vi "uA_Measurement_kit_Logging.vi"() -> ()   [LabVIEW 2017]
uses:
  Range_Shunt_selector.ctl
  <vilib>/Waveform/WDTFileIO.llb/ Write Waveform to File.vi
  <vilib>/Utility/file.llb/Write Delimited Spreadsheet (string).vi
  <vilib>/Waveform/WDTFileIO.llb/Read Waveform from File.vi
  <vilib>/Utility/config.llb/Write Key (I32).vi
  <vilib>/Utility/config.llb/Write Key (Boolean).vi
  <vilib>/Utility/config.llb/Read Key (I32).vi
  <vilib>/Utility/config.llb/Read Key (Boolean).vi
  <vilib>/measure/madcrms.llb/Basic Averaged DC-RMS for 1 Chan.vi
  <resource>/objmgr/daqmx.rc
  <vilib>/Utility/config.llb/NI_LVConfig.lvlib
  <vilib>/measure/NI_MAPro.lvlib
panel:
  out "First_time":timestamp
  out "Ver":string
  out "appended path":path
  out "current time":timestamp
  out "Samples":i32=20000
  out "error out 3":errorcluster
  out "PhysicalChanName":tag
  out "DEV SN":u32 format="%.0x"
  out "mARange":dbl
  out "Boolean":bool
  out "DevSerialNum":u32
  in  "uA_bank0":dbl=1.5 format="%#_13g"
  out "Task out":refnum<k21>="Stop"
  out "Sample rate":dbl=20000.0 format="%#_13g"
  out "Clear":bool=TRUE
  out "seconds since 1Jan1904":timestamp
  in  "Tab Control":enum32{"Current Tracking", "Logging"}(tab)
  out "String":string
  out "Save":bool
  out "Total Time":i32 format="%<%H:%M:%S>t "
  in  "Sampling Rate":T1(ring)
  out "out_range":bool
  in  "Save setting":bool
  out "PW_Source":bool
  out "EX_IN_INdicator":bool
  out "Lable.Unit_VOl_MA_UA":string
  in  "Ext PW Vol Monitor":bool
  out "POWER ON_OFF":bool
  out "vbat_lb":dbl format="%#_4f"
  in  "bypass Shunt":bool
  in  "Internal PW":bool
  in  "USB":tag="Dev1"
  out "schematic":bool
  in  "Save":bool
  in  "Load":bool
  in  "Calib":bool
  in  "Power ON/OFF":bool
  in  "Profile":enum16{"SAM", "DIANA", "Hi-POWER", "Other..."}(ring)
  in  "Take Picture":bool
  in  "Orginal":bool
  in  "Clear Graph":bool
  in  "ZOOM M1M2":bool
  in  "ZOOM -":bool
  in  "ZOOM +":bool
  in  "stop":bool
  out "Vbat":dbl format="%#.3f"
  in  "Measure":bool
  in  "Range - Shunts":T2
  out "PW_Internal_Source":dbl
  out "Min":dbl
  out "Max":dbl
  out "Delta(s)":sgl
  in  "Center":bool
  out "Avg":dbl
  out "Waveform_main":waveform(sgl)(graph)
  out "Waveform_sub":waveform(dbl)(graph)
  out "Average (uA)":dbl caption="Average (mA)" format="%#_6f"
  in  "Vout  - Vbat profile":enum16{"3.8VDC", "2.9VDC", "By Pass", "4.0VDC"}(ring)=enum."2.9VDC" caption="Vout  - Vbat"
  # "Vbat"
  # "Vdut- Vbat"
  # "DUT"
  # "µPower kit for Wear OS Dev"
  # "Rs"
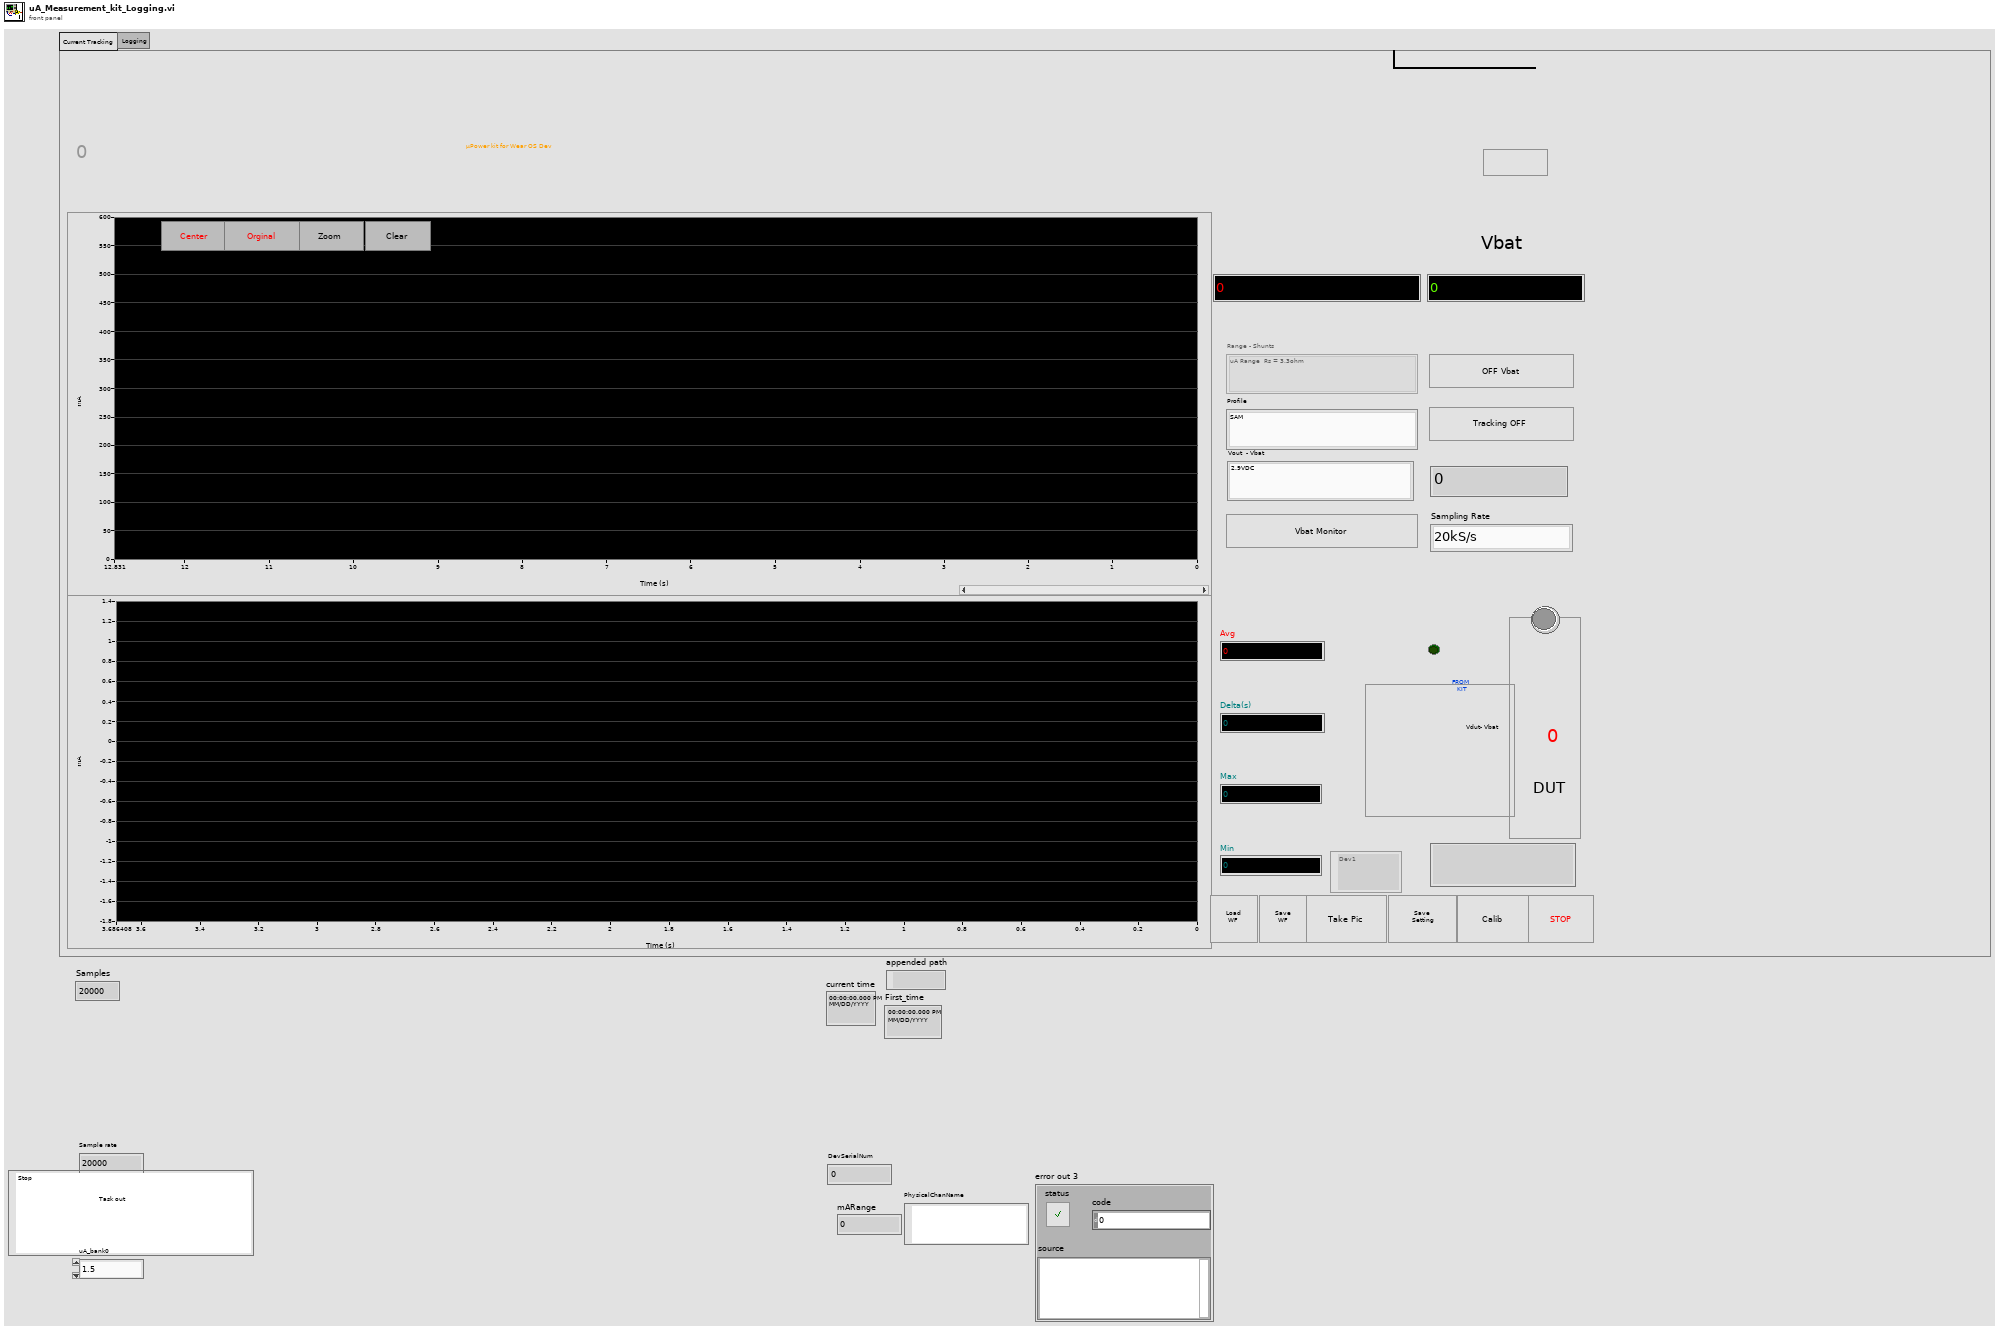
[diagram p1: front panel]
types:
  T1 = enum16{"20kS/s", "10kS/s", "5kS/s", "2kS/s", "1kS/s", "500S/s", "100S/s"}
  T2 = typedef "Range_Shunt_selector.ctl" = enum16{"uA Range  Rs = 3.3ohm", "mA Range Rs = 3.3ohm", "mA Range Rs = 1ohm", "mA Range Rs = 1ohm - X2"}
  T3 = enum8{"Enabled", "Disabled", "Disabled and Grayed Out"}
  T4 = enum16{"open", "replace", "create", "open or create", "replace or create", "replace or create with confirmation"}
  T5 = typedef "NI_LVConfig.lvlib/Config Data RefNum.ctl" = refnum<k1>
  T6 = enum16{"Internal PW Source", "External PW Source"}
  T7 = enum16{"Turn On bypass - Off Shunt", "Turn Off bypass - On Shunt"}
  T8 = typedef "LVCursorListTypeDef.ctl" = cluster{"Name":string, "Color":u32, "Style":u8, "Point Style":u8, "Name Visible":bool, "Allow Drag":bool, "Cursor Mode":u32, "Plot":i32, "Index":i32, "Position":cluster{"X":dbl, "Y":dbl}, "X Scale":u32, "Y Scale":u32, "Watch Plots":i32[], "Watch All Plots":bool, "Plot Area":i32, "Label Offset":cluster{"X":dbl, "Y":dbl}}[]
  T9 = typedef "imagedata.ctl" = cluster{"image type":i32, "image depth":i32, "image":u8[], "mask":u8[], "colors":u32[], "Rectangle":cluster{"left":i16, "top":i16, "right":i16, "bottom":i16}}
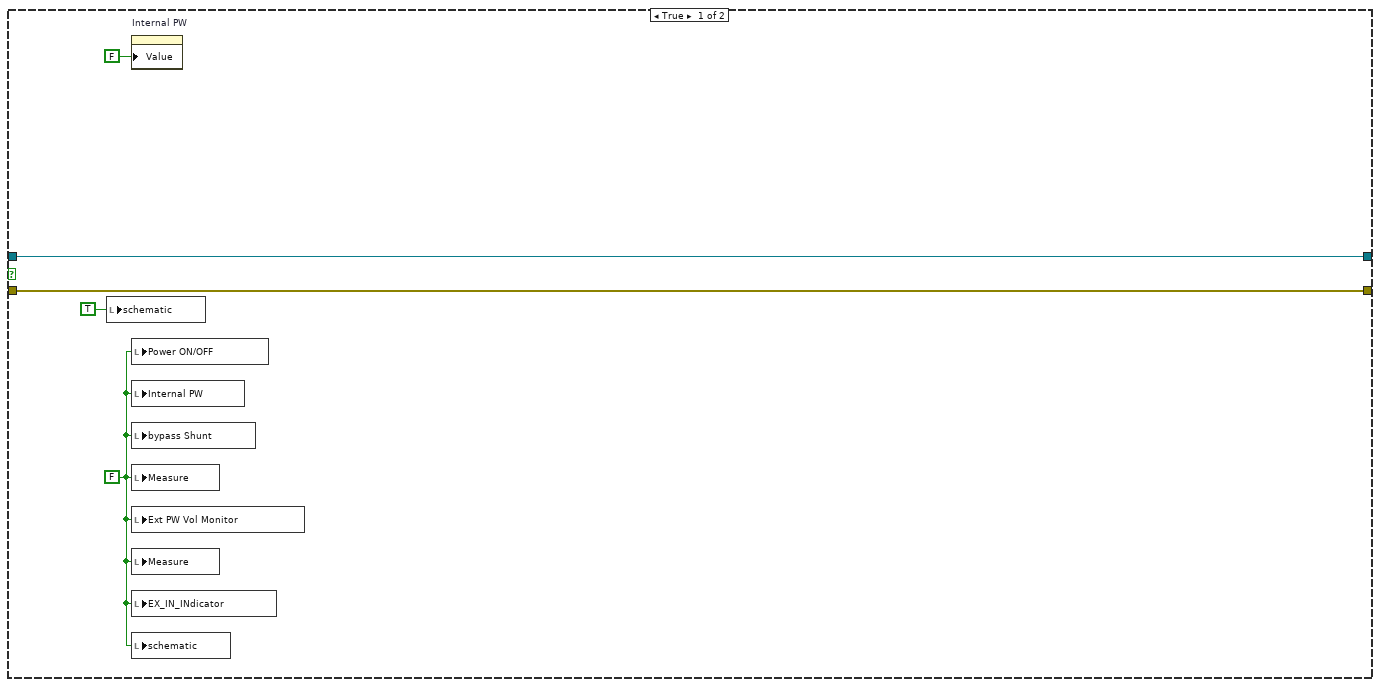
[diagram p3: hidden frame]
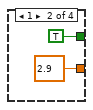
[diagram p4: hidden frame]
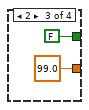
[diagram p5: hidden frame]
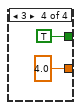
[diagram p6: hidden frame]
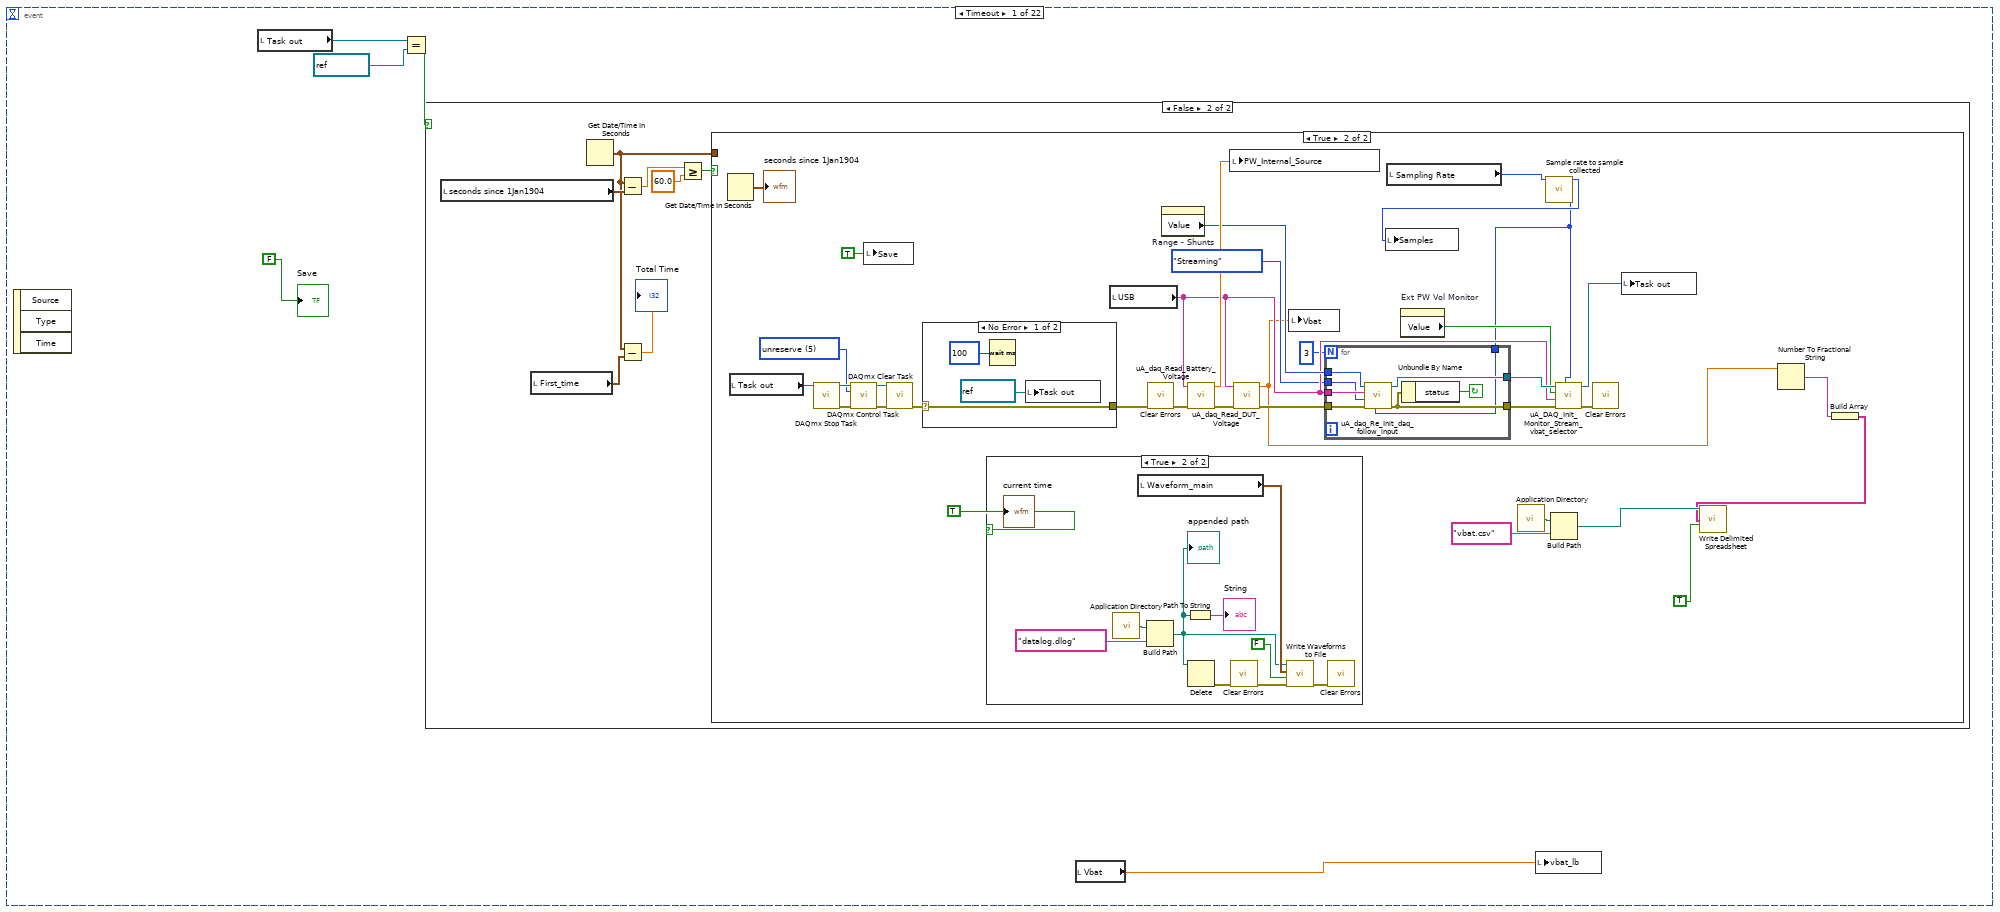
[diagram p8: hidden frame]
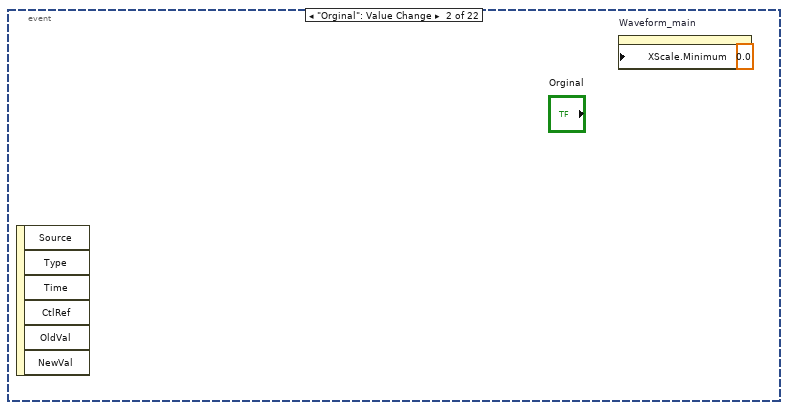
[diagram p13: hidden frame]
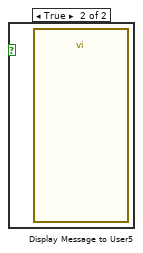
[diagram p14: hidden frame]
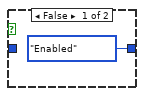
[diagram p15: hidden frame]
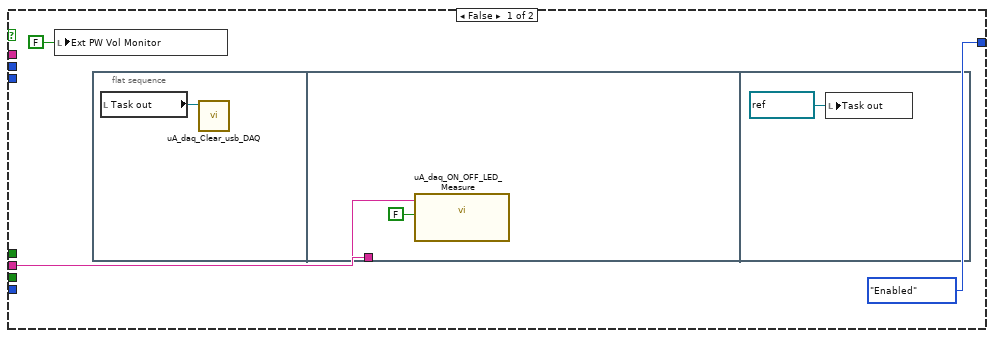
[diagram p16: hidden frame]
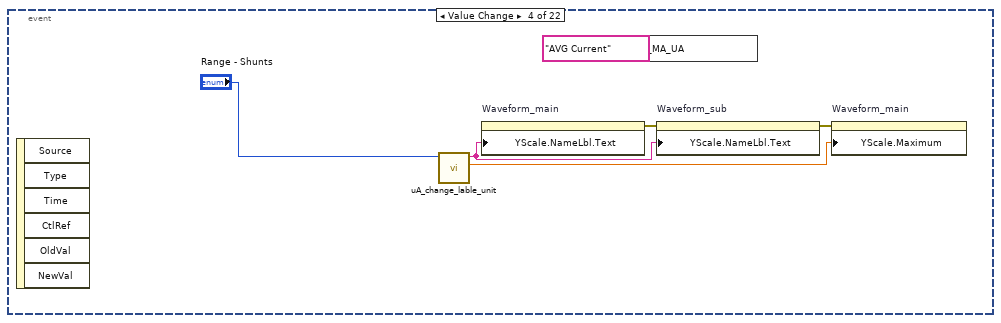
[diagram p17: hidden frame]
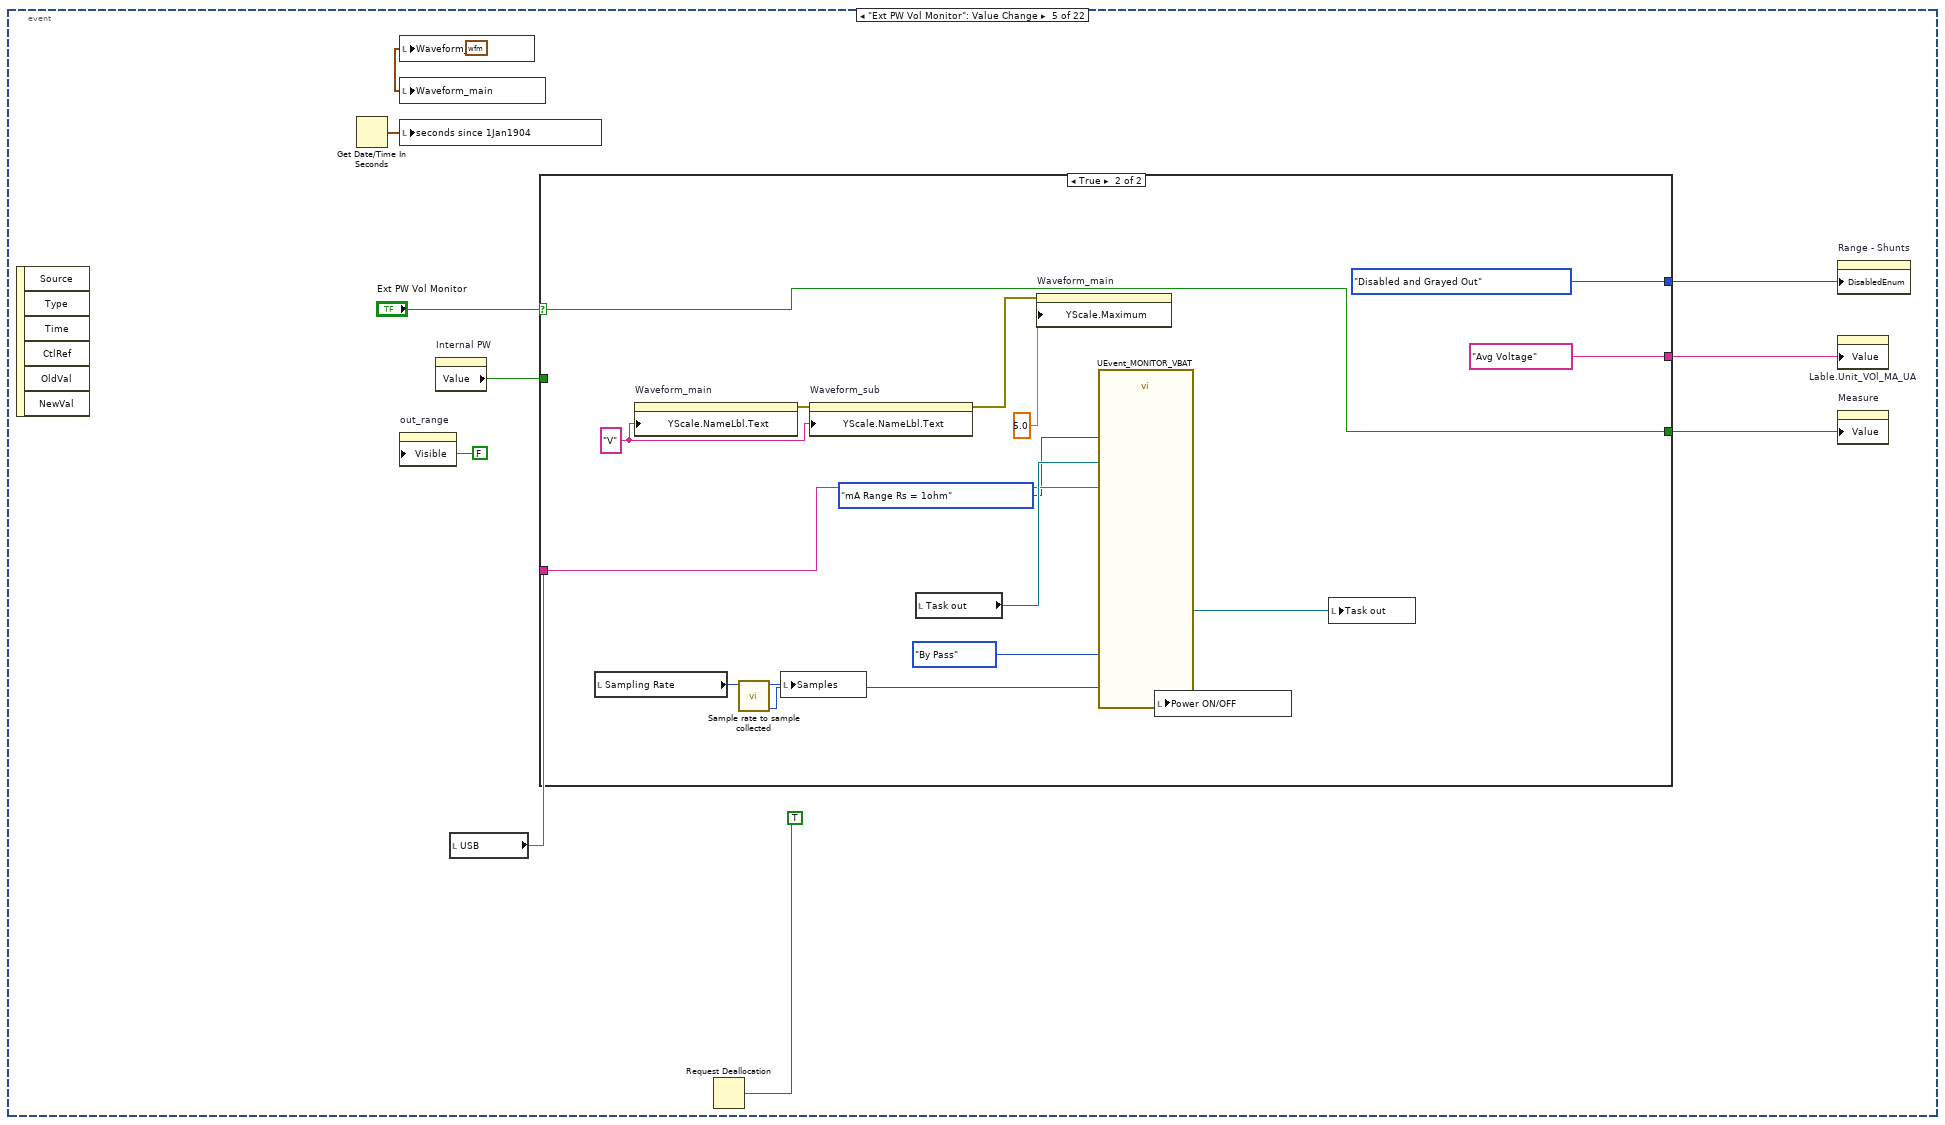
[diagram p18: hidden frame]
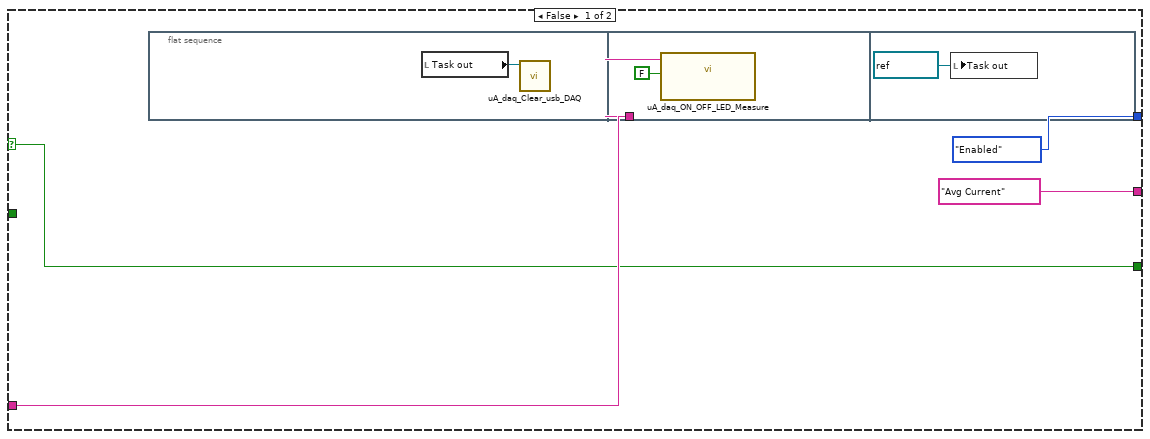
[diagram p19: hidden frame]
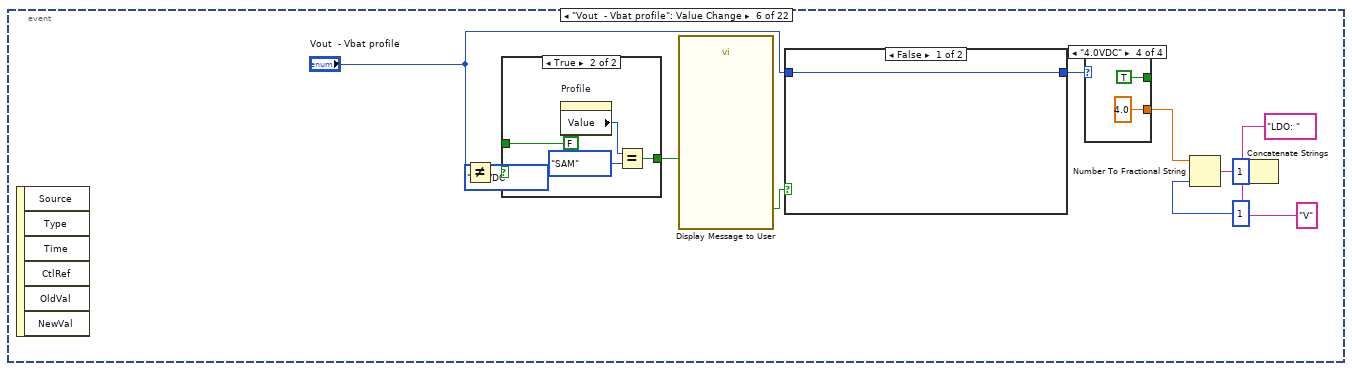
[diagram p20: hidden frame]
diagram:
  w2 = 24164516  # 1200s
  n1 = flat-sequence {
    tunnel: [w45] -> w5
    tunnel: [w48] -> w4
    frame #0 {
      w15 = TRUE ("s")
      w26 = FALSE ("Power ON/OFF")
      w45 = refnum<k21> "Stop" ("task out")
      n2 = property class="DAQmx System"() -> (error out=w39:errorcluster, "Device Names"=w40:tag[])  [unwired: 2 in, 1 out]
      n3 = property on="Range - Shunts" class="Enum (strict)"("DisabledEnum"=T3."Enabled" ("Disabled")) -> (error out=w8:errorcluster)  [unwired: 2 in, 1 out]
      n4 = local write "Vout  - Vbat profile"(enum16{"3.8VDC", "2.9VDC", "By Pass", "4.0VDC"}."By Pass" ("Vout  - Vbat profile")) -> ()
      n5 = local write "Profile"(enum16{"SAM", "DIANA", "Hi-POWER", "Other..."}."Hi-POWER" ("Profile")) -> ()
      n6 = for {
        tunnel: w40 -> [w102] mode=indexing
        shift-right: [w106] -> _
        shift-left: w39 -> [w107]
        tunnel: [w102] -> w38
        tunnel: [w101] -> w20
        stop <- w103 stop-if-true
        n7 = property class="DAQmx Device"(error in=w107, "Active Device"=w102) -> (error out=w106:errorcluster, "DevSerialNum"=w101:u32, "DevIsSimulated"=w105:bool)  [unwired: 1 in, 1 out]
        n8 = Equal?(x=w105, y=FALSE) -> (x = y?=w103:bool)
      }
      "DEV SN" <- w20
      n9 = local write "Power ON/OFF"(w26) -> ()
      n10 = local write "POWER ON_OFF"(w26) -> ()
      n11 = Select(t="Average (mA)" ("Caption.Text"), s=w15, f="Average (uA)" ("Caption.Text")) -> (s? t:f=w18:string)
      n12 = call <vilib>:"Application Directory.vi"() -> ("Application Directory"=w33:path)
      n13 = Select(t="mA" ("Caption.Text"), s=w15, f="uA" ("Caption.Text")) -> (s? t:f=w17:string)
      n14 = property on="out_range" class="Bool (strict)"(error in=w8, "Visible"=FALSE) -> (error out=w11:errorcluster)  [unwired: 1 in, 1 out]
      n15 = Build Path(base path=w33, name or relative path="Setting.cfg") -> (appended path=w31:path)
      n16 = property on="Average (uA)" class="DigNum (strict)"("Caption.Text"=w18) -> ()  [unwired: 2 in, 2 out]
      n17 = property on="Waveform_sub" class="WFGraph (strict)"("YScale.NameLbl.Text"=w17) -> ()  [unwired: 2 in, 2 out]
      n18 = property on="Waveform_main" class="WFGraph (strict)"("YScale.NameLbl.Text"=w17) -> ()  [unwired: 2 in, 2 out]
      n19 = call <vilib>:"Open Config Data.vi"("configuration file path"=w31) -> ("error out"=w27:errorcluster, "file created?"=w34:bool, "refnum"=w30:T5)  [unwired: 8 in]
      n20 = property on="Ext PW Vol Monitor" class="Bool (strict)"(error in=w11, "Value"=FALSE ("Record uA & Vbat")) -> (error out=w10:errorcluster)  [unwired: 1 in, 1 out]
      n21 = case shown="False" w34 {
        tunnel: w27 -> [w62 w92]
        tunnel: [w62 w87] -> w28
        tunnel: [w61 w86] -> w29
        tunnel: w30 -> [w61 w75]
        frame True {
          w60 = FALSE ("Measure")
          n22 = local write "schematic"(TRUE ("schematic")) -> ()
          n23 = property on="Internal PW" class="Bool (strict)"("Value"=FALSE ("Internal PW")) -> ()  [unwired: 2 in, 2 out]
          n24 = local write "Power ON/OFF"(w60) -> ()
          n25 = local write "Internal PW"(w60) -> ()
          n26 = local write "bypass Shunt"(w60) -> ()
          n27 = local write "Measure"(w60) -> ()
          n28 = local write "Ext PW Vol Monitor"(w60) -> ()
          n29 = local write "Measure"(w60) -> ()
          n30 = local write "EX_IN_INdicator"(w60) -> ()
          n31 = local write "schematic"(w60) -> ()
        }
        frame False {
          (unwired) FALSE ("Visible")
          w63 = TRUE
          w76 = "SETTING" ("section")
          n32 = Not(x=w63) -> ()  [unwired: 1 out]
          n33 = local write "Internal PW"(w63) -> ()
          n34 = local write "EX_IN_INdicator"(w63) -> ()
          n35 = local write "Vout  - Vbat profile"(enum16{"3.8VDC", "2.9VDC", "By Pass", "4.0VDC"}."By Pass" ("Vout  - Vbat profile")) -> ()
          n36 = local write "Profile"(enum16{"SAM", "DIANA", "Hi-POWER", "Other..."}."Hi-POWER" ("Profile")) -> ()
          n37 = call-poly <vilib>:"Read Key.vi"("section"=w76, "error in (no error)"=w92, "key"="Range - Shunts", "refnum"=w75) -> ("error out"=w91:errorcluster, "refnum out"=w78:T5)  [unwired: 4 in, 2 out]
          n38 = local write "Range - Shunts"(Range_Shunt_selector."mA Range Rs = 1ohm" ("Range - Shunts")) -> ()
          n39 = call-poly <vilib>:"Read Key.vi"("section"=w76, "error in (no error)"=w91, "key"="Profile", "refnum"=w78) -> ("error out"=w90:errorcluster, "refnum out"=w77:T5)  [unwired: 4 in, 2 out]
          n40 = call-poly <vilib>:"Read Key.vi"("section"=w76, "error in (no error)"=w90, "key"="Vout  - Vbat profile", "refnum"=w77) -> ("error out"=w89:errorcluster, "value"=w67:i32, "refnum out"=w79:T5)  [unwired: 4 in, 1 out]
          n41 = case shown="0, Default" w67 {
            tunnel: [3.8 2.9 99.0 4.0] -> w71
            tunnel: [TRUE ("Visible") TRUE ("Visible") FALSE ("Visible") TRUE ("Visible")] -> _
            frame 0, Default {
            }
            frame 1 {
            }
            frame 2 {
            }
            frame 3 {
            }
          }
          n42 = call-poly <vilib>:"Read Key.vi"("section"=w76, "error in (no error)"=w89, "key"="Internal PW", "refnum"=w79) -> ("error out"=w88:errorcluster, "refnum out"=w80:T5)  [unwired: 4 in, 2 out]
          n43 = call-poly <vilib>:"Read Key.vi"("section"=w76, "error in (no error)"=w88, "key"="bypass Shunt", "refnum"=w80) -> ("error out"=w87:errorcluster, "value"=w74:bool, "refnum out"=w86:T5)  [unwired: 4 in, 1 out]
          n44 = local write "bypass Shunt"(w74) -> ()
          n45 = Number To Fractional String(number=w71, width (-)=i16 1, precision (6)=i16 1) -> (F-format string=w68:string)  [unwired: 1 in]
          n46 = Concatenate Strings("LDO: " ("string"), w68, "V" ("string")) -> ()  [unwired: 1 out]
        }
      }
      n47 = local write "USB"(w38) -> ()
      n48 = property on="out_range" class="Bool (strict)"(error in=w10, "Visible"=FALSE) -> (error out=w9:errorcluster)  [unwired: 1 in, 1 out]
      n49 = call "Calibration_load_file.vi"("DEV SN"=w20) -> ("Calib value-mA"=→"mARange":dbl, "Calib value-uA"=w21:dbl)  [unwired: 8 in]
      n50 = local write "uA_bank0"(w21) -> ()
      n51 = call <vilib>:"Application Directory.vi"() -> ("Application Directory"=w47:path)
      n52 = call "uA_build_version.vi"("error in (no error)"=w9, "name or relative path"="uPower_kit_wear_os.exe", "path"=w47) -> ("error out"=w44:errorcluster, "FileVersion"=w43:string)  [unwired: 6 in, 1 out]
      n53 = case shown="Error" w44 {
        selector: w44 -> [_ w110]
        tunnel: w43 -> [w108 _]
        tunnel: [w108 "" ("FileVersion")] -> w42
        frame No Error {
        }
        frame Error {
          n54 = call <vilib>:"Clear Errors.vi"("error in (no error)"=w110) -> ()  [unwired: 5 in, 2 out]
        }
      }
      "Ver" <- w42
      n55 = local write "Measure"(FALSE ("Measure")) -> ()
      n56 = local write "schematic"(TRUE ("schematic")) -> ()
      n57 = disable-structure shown="Disabled" {
        frame Disabled {
          n58 = call <vilib>:"Application Directory.vi"() -> ("Application Directory"=w57:path)
          n59 = Build Path(base path=w57, name or relative path="datalog.dlog" ("pattern label")) -> (appended path=w55:path)
          n60 = Open/Create/Replace File(file path (use dialog)=w55, operation (0:open)=T4."replace or create", access (0:read/write)=enum16{"read/write", "read-only", "write-only"}."write-only") -> ()  [unwired: 3 in, 3 out]
        }
        frame Enabled {
        }
      }
      n61 = call <vilib>:"Close Config Data.vi"("error in (no error)"=w28, "refnum"=w29) -> ()  [unwired: 8 in, 2 out]
      n62 = Obtain Queue(name (unnamed)="Data", element data type=waveform(sgl) {"t0"=timestamp(0 s since 1904-01-01), "dt"=1.0, "Y"=[]} ("Waveform Chart 2")) -> (queue out=w48:refnum<queue>)  [unwired: 3 in, 2 out]
      "Clear" <- FALSE ("Clear")
      "Sample rate" <- 20000.0 ("Sample rate")
      "Task out" <- w45
    }
  }
  n63 = Multiply(x=w2, y=4) -> (x*y=w1:i32)
  n64 = while {
    stop <- FALSE stop-if-true
    n65 = event shown="[2] \"Measure\": Value Change" {
      selector: _ -> [_ _ _ _ _ _ _ _ _ _ _ _ _ _ _ _ _ _ _ _ _ _]
      dyn-events: _ -> [_ _ _ _ _ _ _ _ _ _ _ _ _ _ _ _ _ _ _ _ _ _]
      timeout: 400 -> [_ _ _ _ _ _ _ _ _ _ _ _ _ _ _ _ _ _ _ _ _ _]
      event Timeout {
        n66 = event-data() -> ()  [unwired: 1 in, 3 out]
        n67 = local read "Task out"() -> (w113:refnum<k21>)
        n68 = Equal?(x=w113, y=refnum<k21> "Stop") -> (x = y?=w114:bool)
        n69 = case shown="False" w114 {
          frame True {
          }
          frame False {
            n70 = local read "seconds since 1Jan1904"() -> (w121:timestamp)
            n71 = local read "First_time"() -> (w119:timestamp)
            n72 = Get Date/Time In Seconds() -> (seconds since 1Jan1904=w120:timestamp)
            n73 = Subtract(x=w120, y=w121) -> (x-y=w124:dbl)
            n74 = Subtract(x=w120, y=w119) -> (x-y=→"Total Time":dbl)
            n75 = Greater Or Equal?(x=w124, y=60.0) -> (x >= y?=w122:bool)
            n76 = case shown="True" w122 {
              tunnel: w120 -> [_ _]
              frame False {
              }
              frame True {
                w143 = 5 items=["verify"=2, "reserve"=4, "commit"=3, "unreserve"=5, "abort"=6] ("action")
                n77 = Get Date/Time In Seconds() -> (seconds since 1Jan1904=→"seconds since 1Jan1904":timestamp)
                n78 = local read "Task out"() -> (w157:refnum<k21>)
                n79 = call <vilib>:"DAQmx Stop Task.vi"("task/channels in"=w157) -> ("task out"=w147:refnum<k21>, "error out"=w145:errorcluster)  [unwired: 13 in]
                n80 = call <vilib>:"DAQmx Control Task.vi"("task/channels in"=w147, "action"=w143, "error in"=w145) -> ("task out"=w146:refnum<k21>, "error out"=w144:errorcluster)  [unwired: 11 in]
                n81 = local write "Save"(TRUE ("Save")) -> ()
                n82 = call <vilib>:"DAQmx Clear Task.vi"("task in"=w146, "error in"=w144) -> ("error out"=w139:errorcluster)  [unwired: 13 in]
                n83 = case shown="No Error" w139 {
                  selector: w139 -> [w169 w171]
                  tunnel: [w169 w171] -> w138
                  frame No Error {
                    n84 = Wait (ms)(milliseconds to wait=u32 100) -> ()  [unwired: 1 out]
                    n85 = local write "Task out"(refnum<k21> "Stop" ("Task out")) -> ()
                  }
                  frame Error {
                  }
                }
                n86 = case shown="True" TRUE {
                  frame False {
                  }
                  frame True {
                    n87 = call <vilib>:"Application Directory.vi"() -> ("Application Directory"=w167:path)
                    n88 = local read "Waveform_main"() -> (w164:waveform(sgl))
                    n89 = Build Path(base path=w167, name or relative path="datalog.dlog" ("pattern label")) -> (appended path=w160:path)
                    "appended path" <- w160
                    n90 = Path To String(path=w160) -> (string=→"String":string)
                    n91 = Delete(path (use dialog)=w160) -> (error out=w162:errorcluster)  [unwired: 4 in, 2 out]
                    n92 = call <vilib>:"Clear Errors.vi"("error in (no error)"=w162) -> ("error out"=w161:errorcluster)  [unwired: 5 in, 1 out]
                    n93 = call-poly <vilib>:"Write Waveforms to File.vi"("error in (no error)"=w161, "append to file? (new file:F)"=FALSE, "waveform"=w164, "file path (dialog if empty)"=w160) -> ("error out"=w163:errorcluster)  [unwired: 6 in, 1 out]
                    n94 = call <vilib>:"Clear Errors.vi"("error in (no error)"=w163) -> ()  [unwired: 5 in, 2 out]
                  }
                }
                n95 = local read "USB"() -> (w149:tag)
                n96 = call <vilib>:"Clear Errors.vi"("error in (no error)"=w138) -> ("error out"=w156:errorcluster)  [unwired: 5 in, 1 out]
                n97 = property on="Range - Shunts" class="Enum (strict)"() -> ("Value"=w153:T2)  [unwired: 2 in, 2 out]
                n98 = call "uA_daq_Read_Battery_Voltage.vi"("error in"=w156, "USB DAQ"=w149) -> ("error out"=w154:errorcluster, "Battery_Voltage"=w155:dbl)  [unwired: 8 in]
                n99 = local write "PW_Internal_Source"(w155) -> ()
                n100 = call "uA_daq_Read_DUT_Voltage.vi"("error in"=w154, "USB DAQ"=w149) -> ("error out"=w142:errorcluster, "DUT_Voltage"=w127:dbl)  [unwired: 8 in]
                n101 = local write "Vbat"(w127) -> ()
                n102 = local read "Sampling Rate"() -> (w135:T1)
                n103 = property on="Ext PW Vol Monitor" class="Bool (strict)"() -> ("Value"=w150:bool)  [unwired: 2 in, 2 out]
                n104 = call <vilib>:"Application Directory.vi"() -> ("Application Directory"=w130:path)
                n105 = call "Sample rate to sample collected.vi"("Sampling Rate _menu"=w135) -> ("Sample_rate"=w134:u32, "Sample"=w136:i32)  [unwired: 9 in]
                n106 = for {
                  N: 3 -> [_]
                  tunnel: w153 -> [w179]
                  tunnel: [w178] -> w152
                  tunnel: w149 -> [w177]
                  tunnel: enum16{"Streaming", "Read All", "Stop"}."Streaming" ("Acquire Mode") -> [w175]
                  tunnel: w142 -> [w176]
                  tunnel: [w174] -> w148
                  tunnel: w134 -> [w172]
                  stop <- w173 continue-if-true
                  n107 = call "uA_daq_Re_Init_daq_follow_input.vi"("rate"=w172, "error in (no error)"=w176, "Acquire Mode"=w175, "USB"=w177, "Range_shunt"=w179) -> ("error out"=w174:errorcluster, "Refnum out"=w178:refnum<k21>)  [unwired: 5 in]
                  n108 = Unbundle By Name(w174) -> ("status"=w173:bool)
                }
                n109 = local write "Samples"(w136) -> ()
                n110 = Build Path(base path=w130, name or relative path="vbat.csv" ("pattern label")) -> (appended path=w129:path)
                n111 = call "uA_DAQ_Init_Monitor_Stream_vbat_selector.vi"("Sample rate"=w134, "error in (no error)"=w148, "USB"=w149, "Ext PW Vol Monitor"=w150, "Refnum in"=w152) -> ("error out"=w137:errorcluster, "Refnum out"=w151:refnum<k21>)  [unwired: 5 in]
                n112 = call <vilib>:"Clear Errors.vi"("error in (no error)"=w137) -> ()  [unwired: 5 in, 2 out]
                n113 = local write "Task out"(w151) -> ()
                n114 = Number To Fractional String(number=w127) -> (F-format string=w126:string)  [unwired: 3 in]
                n115 = Build Array(w126) -> (w125:string[])
                n116 = call-poly <vilib>:"Write Delimited Spreadsheet.vi"("file path (dialog if empty)"=w129, "1D data"=w125, "append to file? (new file:F)"=TRUE) -> ()  [unwired: 11 in, 2 out]
              }
            }
          }
        }
        n117 = local read "Vbat"() -> (w117:dbl)
        n118 = local write "vbat_lb"(w117) -> ()
        "Save" <- FALSE ("Save")
      }
      event "Orginal": Value Change {
        n119 = event-data() -> ()  [unwired: 1 in, 6 out]
        n120 = property on="Waveform_main" class="WFGraph (strict)"("XScale.Minimum"=0.0 ("X Scale.Range:Minimum")) -> ()  [unwired: 2 in, 2 out]
      }
      event "Measure": Value Change {
        (unwired) Range_Shunt_selector."uA Range  Rs = 3.3ohm" ("Range - Shunts")
        n121 = event-data() -> ()  [unwired: 1 in, 6 out]
        n122 = Get Date/Time In Seconds() -> (seconds since 1Jan1904=w205:timestamp)
        n123 = local read "DEV SN"() -> (w187:u32)
        n124 = local write "seconds since 1Jan1904"(w205) -> ()
        n125 = local read "Vout  - Vbat profile"() -> (w202:enum16{"3.8VDC", "2.9VDC", "By Pass", "4.0VDC"})
        n126 = property on="Ext PW Vol Monitor" class="Bool (strict)"() -> ("Value"=w195:bool)  [unwired: 2 in, 2 out]
        n127 = property on="Vout  - Vbat profile" class="Enum (strict)"() -> ("RingText.Text"=w203:string)  [unwired: 2 in, 2 out]
        n128 = local read "Range - Shunts"() -> (w193:T2)
        n129 = call "Calibration_load_file.vi"("DEV SN"=w187) -> ("Calib value-uA"=w186:dbl)  [unwired: 8 in, 1 out]
        n130 = Equal To 0?(x=w186) -> (x = 0?=w185:bool)
        n131 = property on="Internal PW" class="Bool (strict)"() -> ("Value"=w196:bool)  [unwired: 2 in, 2 out]
        n132 = local write "Lable.Unit_VOl_MA_UA"("Avg Current" ("Lable.Unit_VOl_MA_UA")) -> ()
        n133 = case shown="False" w185 {
          frame False {
          }
          frame True {
            n134 = call "Display Message to User5"() -> ()  [unwired: 10 in, 2 out]
          }
        }
        n135 = local read "Profile"() -> (w201:enum16{"SAM", "DIANA", "Hi-POWER", "Other..."})
        n136 = case shown="True" "Measure" {
          tunnel: w203 -> [_ _]
          tunnel: w202 -> [_ _]
          tunnel: w201 -> [_ _]
          tunnel: w193 -> [_ w232]
          tunnel: w196 -> [_ w228]
          tunnel: "USB" -> [w210 w226]
          tunnel: w195 -> [_ w223]
          tunnel: [T3."Enabled" ("Disabled") T3."Disabled and Grayed Out" ("Disabled")] -> w189
          frame False {
            n137 = local write "Ext PW Vol Monitor"(FALSE ("Ext PW Vol Monitor")) -> ()
            n138 = flat-sequence {
              tunnel: w210 -> [w214]
              frame #0 {
                n139 = local read "Task out"() -> (w212:refnum<k21>)
                n140 = call "uA_daq_Clear_usb_DAQ.vi"("Refnum in"=w212) -> ()  [unwired: 11 in]
              }
              frame #1 {
                n141 = call "uA_daq_ON_OFF_LED_Measure.vi"("LED_meas"=FALSE ("Boolean"), "USB"=w214) -> ()  [unwired: 9 in, 1 out]
              }
              frame #2 {
                n142 = local write "Task out"(refnum<k21> "Stop" ("Refnum out")) -> ()
              }
            }
          }
          frame True {
            n143 = local write "Ext PW Vol Monitor"(FALSE ("Ext PW Vol Monitor")) -> ()
            n144 = property on="Vout  - Vbat profile" class="Enum (strict)"() -> ("Value"=w229:enum16{"3.8VDC", "2.9VDC", "By Pass", "4.0VDC"})  [unwired: 2 in, 2 out]
            n145 = local read "Task out"() -> (w231:refnum<k21>)
            n146 = Get Date/Time In Seconds() -> (seconds since 1Jan1904=→"First_time":timestamp)
            n147 = call "Sample rate to sample collected.vi"("Sampling Rate _menu"="Sampling Rate") -> ("Sample_rate"=w217:u32, "Sample"=→"Samples":i32)  [unwired: 9 in]
            n148 = call "UEvent_MEASURE_FULL_PROCESS_START.vi"("Refnum in"=w231, "Range - Shunts"=w232, "Ext PW Vol Monitor"=w223, "USB"=w226, "Internal/external Power"=w228, "Vout  - Vbat profile"=w229, "Sample rate"=w217) -> ("DevSerialNum"=→"DevSerialNum":u32, "Power ON/OFF"=w234:bool, "Refnum out"=w225:refnum<k21>, "Battery_Voltage"=→"PW_Internal_Source":dbl, "DUT_Voltage"=→"Vbat" →"vbat_lb":dbl, "Measure indicator"=w227:bool)  [unwired: 2 in, 1 out]
            n149 = property on="Power ON/OFF" class="Bool (strict)"("Value"=w227) -> ()  [unwired: 2 in, 2 out]
            n150 = property on="Measure" class="Bool (strict)"("Value"=w227) -> ()  [unwired: 2 in, 2 out]
            n151 = local write "Power ON/OFF"(w234) -> ()
            n152 = property class="DAQmx Channel"(reference=w225) -> (error out=w222:errorcluster, "PhysicalChanName"=→"PhysicalChanName":tag)  [unwired: 1 in, 1 out]
            n153 = local write "Task out"(w225) -> ()
            n154 = call <vilib>:"Clear Errors.vi"("error in (no error)"=w222) -> ()  [unwired: 5 in, 2 out]
          }
        }
        n155 = call "uA_change_lable_unit.vi"("Range - Shunts"=w193) -> ("Y_scale"=w198:dbl, "unit"=w197:string)  [unwired: 8 in, 1 out]
        n156 = property on="Waveform_main" class="WFGraph (strict)"("YScale.NameLbl.Text"=w197) -> (error out=w200:errorcluster)  [unwired: 2 in, 1 out]
        n157 = property on="Waveform_sub" class="WFGraph (strict)"(error in=w200, "YScale.NameLbl.Text"=w197) -> (error out=w199:errorcluster)  [unwired: 1 in, 1 out]
        n158 = property on="Waveform_main" class="WFGraph (strict)"(error in=w199, "YScale.Maximum"=w198) -> ()  [unwired: 1 in, 2 out]
        n159 = Request Deallocation(TRUE ("flag")) -> ()
        n160 = call <vilib>:"Application Directory.vi"() -> ("Application Directory"=w184:path)
        n161 = Build Path(base path=w184, name or relative path="vbat.csv" ("pattern label")) -> (appended path=w182:path)
        n162 = Delete(path (use dialog)=w182) -> (error out=w181:errorcluster)  [unwired: 4 in, 2 out]
        n163 = call <vilib>:"Clear Errors.vi"("error in (no error)"=w181) -> ()  [unwired: 5 in, 2 out]
        n164 = property on="Range - Shunts" class="Enum (strict)"("DisabledEnum"=w189) -> (error out=w192:errorcluster)  [unwired: 2 in, 1 out]
        n165 = property on="Measure" class="Bool (strict)"(error in=w192) -> ("Value"=w191:bool)  [unwired: 1 in, 2 out]
        n166 = case shown="True" w191 {
          tunnel: [T3."Enabled" ("Disabled") w208] -> w190
          tunnel: w189 -> [_ w208]
          frame False {
          }
          frame True {
          }
        }
        n167 = property on="Range - Shunts" class="Enum (strict)"("DisabledEnum"=w190) -> ()  [unwired: 2 in, 2 out]
      }
      event Value Change {
        n168 = event-data() -> ()  [unwired: 1 in, 6 out]
        n169 = call "uA_change_lable_unit.vi"("Range - Shunts"="Range - Shunts") -> ("Y_scale"=w239:dbl, "unit"=w238:string)  [unwired: 8 in, 1 out]
        n170 = property on="Waveform_main" class="WFGraph (strict)"("YScale.NameLbl.Text"=w238) -> (error out=w241:errorcluster)  [unwired: 2 in, 1 out]
        n171 = local write "Lable.Unit_VOl_MA_UA"("AVG Current" ("Lable.Unit_VOl_MA_UA")) -> ()
        n172 = property on="Waveform_sub" class="WFGraph (strict)"(error in=w241, "YScale.NameLbl.Text"=w238) -> (error out=w240:errorcluster)  [unwired: 1 in, 1 out]
        n173 = property on="Waveform_main" class="WFGraph (strict)"(error in=w240, "YScale.Maximum"=w239) -> ()  [unwired: 1 in, 2 out]
      }
      event "Ext PW Vol Monitor": Value Change {
        w244 = waveform(sgl) {"t0"=timestamp(0 s since 1904-01-01), "dt"=1.0, "Y"=[]} ("Waveform_main")
        n174 = event-data() -> ()  [unwired: 1 in, 6 out]
        n175 = Get Date/Time In Seconds() -> (seconds since 1Jan1904=w250:timestamp)
        n176 = local write "Waveform_sub"(w244) -> ()
        n177 = local write "Waveform_main"(w244) -> ()
        n178 = local write "seconds since 1Jan1904"(w250) -> ()
        n179 = property on="out_range" class="Bool (strict)"("Visible"=FALSE) -> ()  [unwired: 2 in, 2 out]
        n180 = property on="Internal PW" class="Bool (strict)"() -> ("Value"=w249:bool)  [unwired: 2 in, 2 out]
        n181 = local read "USB"() -> (w247:tag)
        n182 = case shown="True" "Ext PW Vol Monitor" {
          selector: "Ext PW Vol Monitor" -> [w254 w272]
          tunnel: w249 -> [_ _]
          tunnel: w247 -> [w255 w273]
          tunnel: [w254 w272] -> w246
          tunnel: ["Avg Current" ("Lable.Unit_VOl_MA_UA") "Avg Voltage" ("Lable.Unit_VOl_MA_UA")] -> w245
          tunnel: [T3."Enabled" ("Disabled") T3."Disabled and Grayed Out" ("Disabled")] -> w243
          frame False {
            n183 = flat-sequence {
              tunnel: w255 -> [w258]
              frame #0 {
                n184 = local read "Task out"() -> (w256:refnum<k21>)
                n185 = call "uA_daq_Clear_usb_DAQ.vi"("Refnum in"=w256) -> ()  [unwired: 11 in]
              }
              frame #1 {
                n186 = call "uA_daq_ON_OFF_LED_Measure.vi"("LED_meas"=FALSE ("Boolean"), "USB"=w258) -> ()  [unwired: 9 in, 1 out]
              }
              frame #2 {
                n187 = local write "Task out"(refnum<k21> "Stop" ("Refnum out")) -> ()
              }
            }
          }
          frame True {
            w271 = "V" ("Y Scale.Name Label.Text")
            n188 = local read "Sampling Rate"() -> (w263:T1)
            n189 = property on="Waveform_main" class="WFGraph (strict)"("YScale.NameLbl.Text"=w271) -> (error out=w268:errorcluster)  [unwired: 2 in, 1 out]
            n190 = call "Sample rate to sample collected.vi"("Sampling Rate _menu"=w263) -> ("Sample_rate"=w262:u32, "Sample"=w264:i32)  [unwired: 9 in]
            n191 = local write "Samples"(w264) -> ()
            n192 = property on="Waveform_sub" class="WFGraph (strict)"(error in=w268, "YScale.NameLbl.Text"=w271) -> (error out=w269:errorcluster)  [unwired: 1 in, 1 out]
            n193 = local read "Task out"() -> (w274:refnum<k21>)
            n194 = property on="Waveform_main" class="WFGraph (strict)"(error in=w269, "YScale.Maximum"=5.0 ("Y Scale.Range:Maximum")) -> ()  [unwired: 1 in, 2 out]
            n195 = call "UEvent_MONITOR_VBAT.vi"("Vout  - Vbat profile"=enum16{"3.8VDC", "2.9VDC", "By Pass", "4.0VDC"}."By Pass", "Sample rate"=w262, "USB"=w273, "Range - Shunts"=Range_Shunt_selector."mA Range Rs = 1ohm", "Refnum in"=w274) -> ("Refnum out"=w266:refnum<k21>, "Power ON/OFF"=w275:bool)  [unwired: 1 in, 4 out]
            n196 = local write "Power ON/OFF"(w275) -> ()
            n197 = local write "Task out"(w266) -> ()
          }
        }
        n198 = Request Deallocation(TRUE ("flag")) -> ()
        n199 = property on="Range - Shunts" class="Enum (strict)"("DisabledEnum"=w243) -> ()  [unwired: 2 in, 2 out]
        n200 = property on="Lable.Unit_VOl_MA_UA" class="Str"("Value"=w245) -> ()  [unwired: 2 in, 2 out]
        n201 = property on="Measure" class="Bool (strict)"("Value"=w246) -> ()  [unwired: 2 in, 2 out]
      }
      event "Vout  - Vbat profile": Value Change {
        n202 = event-data() -> ()  [unwired: 1 in, 6 out]
        n203 = Not Equal?(x="Vout  - Vbat profile", y=enum16{"3.8VDC", "2.9VDC", "By Pass", "4.0VDC"}."2.9VDC" ("Vout  - Vbat profile")) -> (x != y?=w288:bool)
        n204 = case shown="True" w288 {
          tunnel: [w299 w300] -> w286
          tunnel: FALSE -> [w299 _]
          frame False {
          }
          frame True {
            n205 = property on="Profile" class="Enum (strict)"() -> ("Value"=w302:enum16{"SAM", "DIANA", "Hi-POWER", "Other..."})  [unwired: 2 in, 2 out]
            n206 = Equal?(x=w302, y=enum16{"SAM", "DIANA", "Hi-POWER", "Other..."}."SAM" ("Profile")) -> (x = y?=w300:bool)
          }
        }
        n207 = call "Display Message to User"("Enable"=w286) -> ("OK"=w285:bool)  [unwired: 9 in, 1 out]
        n208 = case shown="False" w285 {
          tunnel: [w297 w298] -> w282
          tunnel: "Vout  - Vbat profile" -> [w297 _]
          frame False {
          }
          frame True {
            w298 = enum16{"3.8VDC", "2.9VDC", "By Pass", "4.0VDC"}."2.9VDC" ("Vout  - Vbat profile")
            n209 = property on="Vout  - Vbat profile" class="Enum (strict)"("Value"=w298) -> ()  [unwired: 2 in, 2 out]
          }
        }
        n210 = case shown="\"4.0VDC\"" w282 {
          tunnel: [3.8 2.9 99.0 4.0] -> w278
          tunnel: [TRUE ("Visible") TRUE ("Visible") FALSE ("Visible") TRUE ("Visible")] -> _
          frame "3.8VDC", Default {
          }
          frame "2.9VDC" {
          }
          frame "By Pass" {
          }
          frame "4.0VDC" {
          }
        }
        n211 = Number To Fractional String(number=w278, width (-)=i16 1, precision (6)=i16 1) -> (F-format string=w281:string)  [unwired: 1 in]
        n212 = Concatenate Strings("LDO: " ("string"), w281, "V" ("string")) -> ()  [unwired: 1 out]
      }
      event "Internal PW": Value Change {
        n213 = event-data() -> ()  [unwired: 1 in, 6 out]
        n214 = local read "Sampling Rate"() -> (w305:T1)
        n215 = case shown="True" "Internal PW" {
          tunnel: [T6."Internal PW Source" ("Ex/Int PW") T6."External PW Source" ("Ex/Int PW")] -> w317
          frame False {
            # "Internal power source"
          }
          frame True {
            # "External Power Source"
          }
        }
        n216 = property on="Ext PW Vol Monitor" class="Bool (strict)"() -> ("Value"=w313:bool)  [unwired: 2 in, 2 out]
        n217 = property on="Range - Shunts" class="Enum (strict)"() -> ("Value"=w316:T2)  [unwired: 2 in, 2 out]
        n218 = local read "Task out"() -> (w320:refnum<k21>)
        n219 = local read "USB"() -> (w315:tag)
        n220 = call "Sample rate to sample collected.vi"("Sampling Rate _menu"=w305) -> ("Sample_rate"=w303:u32, "Sample"=w304:i32)  [unwired: 9 in]
        n221 = local write "Samples"(w304) -> ()
        n222 = call "UEvent_SET_INTERNAL_EXTERNAL_POWER_SOURCE.vi"("Ex/Int PW"=w317, "Sample rate"=w303, "Ext PW Vol Monitor"=w313, "USB"=w315, "Value"=w316, "Refnum in"=w320) -> ("External Voltage HIGH"=w312:bool, "Battery_Voltage"=w319:dbl, "DUT_Voltage"=w318:dbl, "Refnum out"=w314:refnum<k21>)  [unwired: 2 in]
        n223 = local read "Measure"() -> (w311:bool)
        n224 = case shown="True" w312 {
          tunnel: w312 -> [_ w328]
          tunnel: [w327 w328] -> w307
          tunnel: "Internal PW" -> [w327 _]
          frame True {
          }
          frame False {
            n225 = property on="Internal PW" class="Bool (strict)"("Value"=w328) -> ()  [unwired: 2 in, 2 out]
          }
        }
        n226 = local write "PW_Internal_Source"(w319) -> ()
        n227 = local write "Vbat"(w318) -> ()
        n228 = case shown="False" w311 {
          tunnel: w314 -> [_ w326]
          tunnel: [refnum<k21> "Stop" ("Refnum out") w326] -> w310
          frame False {
          }
          frame True {
          }
        }
        n229 = local read "Vout  - Vbat profile"() -> (w308:enum16{"3.8VDC", "2.9VDC", "By Pass", "4.0VDC"})
        n230 = local write "Task out"(w310) -> ()
        n231 = local write "EX_IN_INdicator"(w307) -> ()
        n232 = Not(x=w307) -> (.not. x?=w306:bool)
        n233 = case shown="\"By Pass\"" w308 {
          tunnel: w306 -> [w321 w322 _ w324]
          tunnel: [w321 w322 FALSE w324] -> _
          frame "3.8VDC", Default {
          }
          frame "2.9VDC" {
          }
          frame "By Pass" {
          }
          frame "4.0VDC" {
          }
        }
        "PW_Source" <- "Internal PW"
      }
      event "bypass Shunt": Value Change {
        n234 = event-data() -> ()  [unwired: 1 in, 6 out]
        n235 = Not(x="bypass Shunt") -> (.not. x?=w340:bool)
        n236 = local read "Sampling Rate"() -> (w332:T1)
        n237 = case shown="True" "bypass Shunt" {
          tunnel: [T7."Turn Off bypass - On Shunt" ("Bypass Shunt") T7."Turn On bypass - Off Shunt" ("Bypass Shunt")] -> w344
          frame False {
            # "add Shunt"
          }
          frame True {
            # "No Shunt"
          }
        }
        n238 = property on="schematic" class="Bool (strict)"("Value"=w340) -> ()  [unwired: 2 in, 2 out]
        n239 = property on="Ext PW Vol Monitor" class="Bool (strict)"() -> ("Value"=w338:bool)  [unwired: 2 in, 2 out]
        n240 = local read "Task out"() -> (w341:refnum<k21>)
        n241 = local read "USB"() -> (w343:tag)
        n242 = call "Sample rate to sample collected.vi"("Sampling Rate _menu"=w332) -> ("Sample_rate"=w331:u32, "Sample"=w333:i32)  [unwired: 9 in]
        n243 = local write "Samples"(w333) -> ()
        n244 = property on="Range - Shunts" class="Enum (strict)"() -> ("Value"=w342:T2)  [unwired: 2 in, 2 out]
        n245 = call "UEvent_SET_BYPASS_SHUNT_OR_NOT.vi"("Sample rate"=w331, "Task in"=w341, "Ext PW Vol Monitor"=w338, "USB"=w343, "Bypass Shunt"=w344, "Range_shunt"=w342) -> ("error out"=→"error out 3":errorcluster, "Task out"=w335:refnum<k21>)  [unwired: 4 in]
        n246 = local read "Measure"() -> (w337:bool)
        n247 = local write "Task out"(w335) -> ()
        n248 = case shown="False" w337 {
          tunnel: w335 -> [_ w346]
          tunnel: [refnum<k21> "Stop" ("Refnum out") w346] -> w336
          frame False {
          }
          frame True {
          }
        }
        n249 = local write "Task out"(w336) -> ()
      }
      event "Power ON/OFF": Value Change {
        n250 = event-data() -> ()  [unwired: 1 in, 6 out]
        n251 = case shown="False" "Power ON/OFF" {
          tunnel: [enum16{"Power ON DUT", "Power OFF DUT"}."Power OFF DUT" ("Power ON/OFF DUT") enum16{"Power ON DUT", "Power OFF DUT"}."Power ON DUT" ("Power ON/OFF DUT")] -> w361
          frame False {
          }
          frame True {
            # "ON"
          }
        }
        n252 = local read "Sampling Rate"() -> (w350:T1)
        n253 = local read "Vout  - Vbat profile"() -> (w360:enum16{"3.8VDC", "2.9VDC", "By Pass", "4.0VDC"})
        n254 = property on="Ext PW Vol Monitor" class="Bool (strict)"() -> ("Value"=w356:bool)  [unwired: 2 in, 2 out]
        n255 = property on="Range - Shunts" class="Enum (strict)"() -> ("Value"=w359:T2)  [unwired: 2 in, 2 out]
        n256 = local read "Task out"() -> (w363:refnum<k21>)
        n257 = local read "USB"() -> (w358:tag)
        n258 = call "Sample rate to sample collected.vi"("Sampling Rate _menu"=w350) -> ("Sample_rate"=w349:u32, "Sample"=w351:i32)  [unwired: 9 in]
        n259 = local write "Samples"(w351) -> ()
        n260 = call "UEvent_ON_OFF_POWER_SOURCE.vi"("Sample rate"=w349, "USB"=w358, "Power ON/OFF DUT"=w361, "Ext PW Vol Monitor"=w356, "Value"=w359, "Vout  - Vbat profile"=w360, "Refnum in"=w363) -> ("Battery_Voltage"=w362:dbl, "DUT_Voltage"=w352:dbl, "Refnum out"=w353:refnum<k21>)  [unwired: 2 in]
        n261 = local read "Measure"() -> (w355:bool)
        n262 = local write "PW_Internal_Source"(w362) -> ()
        n263 = local write "Vbat"(w352) -> ()
        n264 = local write "vbat_lb"(w352) -> ()
        n265 = local write "Task out"(w353) -> ()
        n266 = case shown="False" w355 {
          tunnel: w353 -> [_ w365]
          tunnel: [refnum<k21> "Stop" ("Refnum out") w365] -> w354
          frame False {
          }
          frame True {
          }
        }
        n267 = local write "Task out"(w354) -> ()
        "POWER ON_OFF" <- "Power ON/OFF"
      }
      event "Profile": Value Change {
        n268 = event-data() -> ()  [unwired: 1 in, 6 out]
        n269 = case shown="\"Hi-POWER\"" "Profile" {
          tunnel: [enum16{"3.8VDC", "2.9VDC", "By Pass", "4.0VDC"}."2.9VDC" ("DUT Voltage Selector") enum16{"3.8VDC", "2.9VDC", "By Pass", "4.0VDC"}."By Pass" ("DUT Voltage Selector") enum16{"3.8VDC", "2.9VDC", "By Pass", "4.0VDC"}."3.8VDC" ("DUT Voltage Selector") enum16{"3.8VDC", "2.9VDC", "By Pass", "4.0VDC"}."By Pass" ("DUT Voltage Selector")] -> w368
          frame "SAM", Default {
          }
          frame "Other..." {
          }
          frame "DIANA" {
          }
          frame "Hi-POWER" {
          }
        }
        n270 = local write "Vout  - Vbat profile"(w368) -> ()
      }
      event "Waveform_main": Cursor Move {
        n271 = event-data() -> ()  [unwired: 1 in, 9 out]
        n272 = local read "Waveform_main"() -> (w382:waveform(sgl))
        n273 = property on="Waveform_main" class="WFGraph (strict)"() -> ("CrsrList"=w392:T8)  [unwired: 2 in, 2 out]
        n274 = local read "Sampling Rate"() -> (w375:T1)
        n275 = call "Sample rate to sample collected.vi"("Sampling Rate _menu"=w375) -> ("Sample_rate"=w374:u32)  [unwired: 9 in, 1 out]
        n276 = call "uA_daq_Capture_Current_waveform_to_new_chart.vi"("Sample rate"=w374, "CrsrList"=w392, "Waveform_main"=w382) -> ("Numeric"=w389:dbl, "Waveform"=w390:waveform(sgl), "Numeric 2"=w391:sgl)  [unwired: 6 in]
        n277 = local write "Avg"(w391) -> ()
        n278 = local write "Waveform_sub"(w390) -> ()
        n279 = property on="Waveform_sub" class="WFGraph (strict)"("XScale.Maximum"=w389, "XScale.Minimum"=0.0 ("X Scale.Range:Minimum")) -> (error out=w376:errorcluster)  [unwired: 2 in, 1 out]
        n280 = property on="Waveform_main" class="WFGraph (strict)"(error in=w376, "Active Cursor"=u32 1) -> (error out=w384:errorcluster, "Value"=w383:waveform(sgl), "Cursor.Cursor X"=w386:dbl)  [unwired: 1 in, 1 out]
        n281 = property on="Waveform_main" class="WFGraph (strict)" props=["CrsrList", "Active Cursor", "Cursor", "Cursor X"](error in=w384, "Active Cursor"=u32 0) -> ("Cursor.Cursor X"=w385:dbl)  [unwired: 1 in, 3 out]
        n282 = call "uA_daq_calculate_All_values_from Sub_chart.vi"("Cursor.Cursor X 2"=w386, "Cursor.Cursor X"=w385, "Value"=w383, "Sample rate"=w374) -> ("Max value"=→"Max":dbl, "Average"=→"Avg":dbl, "Delta(s)"=→"Delta(s)":sgl, "Min value"=→"Min":dbl)  [unwired: 3 in, 1 out]
      }
      event "Calib": Value Change {
        w398 = Range_Shunt_selector."uA Range  Rs = 3.3ohm" ("Range - Shunts")
        n283 = event-data() -> ()  [unwired: 1 in, 6 out]
        n284 = call "Display Message to User2"() -> ("error out"=w394:errorcluster)  [unwired: 10 in, 1 out]
        n285 = flat-sequence {
          tunnel: w394 -> [_]
          tunnel: [w458] -> w396
          tunnel: [w453] -> w397
          frame #0 {
            n286 = local write "Measure"(FALSE ("Measure")) -> ()
          }
          frame #1 {
            n287 = local read "Task out"() -> (w453:refnum<k21>)
            n288 = local write "Waveform_main"(waveform(sgl) {"t0"=timestamp(0 s since 1904-01-01), "dt"=1.0, "Y"=[]} ("Waveform_main")) -> ()
            n289 = Wait (ms)(milliseconds to wait=u32 1000) -> ()  [unwired: 1 out]
            n290 = local write "uA_bank0"(0.0 ("uA_bank0")) -> ()
            n291 = call <vilib>:"DAQmx Stop Task.vi"("task/channels in"=w453) -> ("task out"=w455:refnum<k21>, "error out"=w456:errorcluster)  [unwired: 13 in]
            n292 = call <vilib>:"DAQmx Clear Task.vi"("task in"=w455, "error in"=w456) -> ("error out"=w454:errorcluster)  [unwired: 13 in]
            n293 = local read "USB"() -> (w458:tag)
            n294 = case shown="Error" w454 {
              frame No Error {
                n295 = local write "Task out"(refnum<k21> "Stop" ("y")) -> ()
              }
              frame Error {
              }
            }
          }
        }
        n296 = call "UEvent_MEASURE_FULL_PROCESS_START.vi"("Refnum in"=w397, "Range - Shunts"=w398, "Ext PW Vol Monitor"=FALSE, "USB"=w396, "Internal/external Power"=FALSE) -> ("Refnum out"=w400:refnum<k21>, "error out"=w401:errorcluster)  [unwired: 4 in, 5 out]
        n297 = while {
          tunnel: w401 -> [w445]
          tunnel: w400 -> [w447]
          tunnel: [w445] -> w399
          stop <- TRUE stop-if-true
          n298 = local write "Task out"(w447) -> ()
          n299 = local write "Measure"(TRUE ("Measure")) -> ()
          n300 = Wait (ms)(milliseconds to wait=u32 10000) -> ()  [unwired: 1 out]
        }
        n301 = flat-sequence {
          tunnel: w399 -> [w440]
          tunnel: w398 -> [w441]
          tunnel: [w440] -> w395
          frame #0 {
            n302 = local read "Average (uA)"() -> (w443:dbl)
            n303 = local read "DEV SN"() -> (w442:u32)
            n304 = local write "Measure"(FALSE ("Measure")) -> ()
            n305 = local write "uA_bank0"(w443) -> ()
            n306 = call "Calibration_Save_file.vi"("Current"=w443, "Range - Shunts"=w441, "DEV SN"=w442) -> ()  [unwired: 8 in, 1 out]
          }
        }
        n307 = flat-sequence {
          tunnel: w395 -> [w410]
          tunnel: [w410] -> w406
          tunnel: [w409] -> w405
          tunnel: [w408] -> w404
          tunnel: [Range_Shunt_selector."mA Range Rs = 1ohm" ("Range - Shunts")] -> w393
          tunnel: w406 -> [_]
          tunnel: w405 -> [w425]
          tunnel: w404 -> [w424]
          tunnel: w393 -> [w422]
          frame #0 {
            n308 = flat-sequence {
              tunnel: [w420] -> w408
              tunnel: [w415] -> w409
              frame #0 {
                n309 = local write "Measure"(FALSE ("Measure")) -> ()
                n310 = Wait (ms)(milliseconds to wait=u32 1000) -> ()  [unwired: 1 out]
              }
              frame #1 {
                n311 = local read "Task out"() -> (w415:refnum<k21>)
                n312 = local read "USB"() -> (w420:tag)
                n313 = local write "Waveform_main"(waveform(sgl) {"t0"=timestamp(0 s since 1904-01-01), "dt"=1.0, "Y"=[]} ("Waveform_main")) -> ()
                n314 = Wait (ms)(milliseconds to wait=u32 2000) -> ()  [unwired: 1 out]
                n315 = local write "mARange"(0.0 ("uA_bank0")) -> ()
                n316 = call <vilib>:"DAQmx Stop Task.vi"("task/channels in"=w415) -> ("task out"=w417:refnum<k21>, "error out"=w418:errorcluster)  [unwired: 13 in]
                n317 = call <vilib>:"DAQmx Clear Task.vi"("task in"=w417, "error in"=w418) -> ("error out"=w416:errorcluster)  [unwired: 13 in]
                n318 = case shown="No Error" w416 {
                  frame No Error {
                    n319 = local write "Task out"(refnum<k21> "Stop" ("y")) -> ()
                  }
                  frame Error {
                  }
                }
              }
            }
          }
          frame #1 {
            n320 = property on="Range - Shunts" class="Enum (strict)"("Value"=w422) -> ()  [unwired: 2 in, 2 out]
            n321 = call "UEvent_MEASURE_FULL_PROCESS_START.vi"("Refnum in"=w425, "Range - Shunts"=w422, "Ext PW Vol Monitor"=FALSE, "USB"=w424, "Internal/external Power"=TRUE) -> ("Refnum out"=w427:refnum<k21>, "error out"=w426:errorcluster)  [unwired: 4 in, 5 out]
            n322 = while {
              tunnel: w426 -> [w435]
              tunnel: w427 -> [w437]
              tunnel: [w435] -> w423
              stop <- TRUE stop-if-true
              n323 = local write "Task out"(w437) -> ()
              n324 = local write "Measure"(TRUE ("Measure")) -> ()
              n325 = Wait (ms)(milliseconds to wait=u32 5000) -> ()  [unwired: 1 out]
            }
            n326 = flat-sequence {
              tunnel: w423 -> [w430]
              tunnel: w422 -> [w431]
              frame #0 {
                n327 = local read "Average (uA)"() -> (w432:dbl)
                n328 = local write "Measure"(FALSE ("Measure")) -> ()
                n329 = local read "DEV SN"() -> (w433:u32)
                n330 = local write "mARange"(w432) -> ()
                n331 = call "Calibration_Save_file.vi"("Current"=w432, "error in (no error)"=w430, "Range - Shunts"=w431, "DEV SN"=w433) -> ()  [unwired: 7 in, 1 out]
              }
            }
          }
          frame #2 {
            n332 = call "Display Message to User3"() -> ()  [unwired: 10 in, 2 out]
          }
        }
      }
      event "Clear Graph": Value Change {
        n333 = event-data() -> ()  [unwired: 1 in, 6 out]
        n334 = flat-sequence {
          frame #0 {
            w460 = waveform(sgl) {"t0"=timestamp(0 s since 1904-01-01), "dt"=1.0, "Y"=[]} ("Waveform_main")
            n335 = local write "Clear"(TRUE ("Clear")) -> ()
            n336 = Wait (ms)(milliseconds to wait=u32 500) -> ()  [unwired: 1 out]
            n337 = local write "Waveform_main"(w460) -> ()
            n338 = local write "Waveform_sub"(w460) -> ()
          }
          frame #1 {
            n339 = local write "Clear"(FALSE ("Clear")) -> ()
          }
        }
      }
      event "ZOOM +": Value Change {
        n340 = event-data() -> ()  [unwired: 1 in, 6 out]
        n341 = property on="Waveform_main" class="WFGraph (strict)" props=["XScale", "Range", "XScale", "Increment", "XScale", "Maximum", "XScale", "Minimum"]() -> ("XScale.Maximum"=w469:dbl, "XScale.Minimum"=w465:dbl)  [unwired: 2 in, 4 out]
        n342 = Subtract(x=w469, y=0.1) -> (x-y=w467:dbl)
        n343 = Add(x=w465, y=0.1) -> (x+y=w464:dbl)
        n344 = property on="Waveform_main" class="WFGraph (strict)"("XScale.Maximum"=w467, "XScale.Minimum"=w464) -> ()  [unwired: 2 in, 2 out]
      }
      event "ZOOM -": Value Change {
        n345 = event-data() -> ()  [unwired: 1 in, 6 out]
        n346 = property on="Waveform_main" class="WFGraph (strict)" props=["XScale", "Range", "XScale", "Increment", "XScale", "Maximum", "XScale", "Minimum"]() -> ("XScale.Maximum"=w478:dbl, "XScale.Minimum"=w474:dbl)  [unwired: 2 in, 4 out]
        n347 = Add(x=w478, y=0.1) -> (x+y=w476:dbl)
        n348 = Subtract(x=w474, y=0.1) -> (x-y=w471:dbl)
        n349 = Less Than 0?(x=w471) -> (x < 0?=w473:bool)
        n350 = Select(t=0.0, s=w473, f=w471) -> (s? t:f=w470:dbl)
        n351 = property on="Waveform_main" class="WFGraph (strict)"("XScale.Maximum"=w476, "XScale.Minimum"=w470) -> ()  [unwired: 2 in, 2 out]
      }
      event "ZOOM M1M2": Value Change {
        n352 = event-data() -> ()  [unwired: 1 in, 6 out]
        n353 = property on="Waveform_main" class="WFGraph (strict)"("Active Cursor"=u32 0) -> (error out=w485:errorcluster)  [unwired: 2 in, 1 out]
        n354 = property on="Waveform_main" class="WFGraph (strict)"(error in=w485) -> (error out=w482:errorcluster, "Cursor.Cursor X"=w480:dbl)  [unwired: 1 in, 1 out]
        n355 = property on="Waveform_main" class="WFGraph (strict)"(error in=w482, "Active Cursor"=u32 1) -> (error out=w484:errorcluster)  [unwired: 1 in, 1 out]
        n356 = property on="Waveform_main" class="WFGraph (strict)"(error in=w484) -> ("Cursor.Cursor X"=w479:dbl)  [unwired: 1 in, 2 out]
        n357 = Greater?(x=w480, y=w479) -> (0:w481:bool)
        n358 = case shown="True" w481 {
          tunnel: w480 -> [w488 w490]
          tunnel: w479 -> [w487 w489]
          frame False {
            n359 = property on="Waveform_main" class="WFGraph (strict)"("XScale.Maximum"=w487, "XScale.Minimum"=w488) -> ()  [unwired: 2 in, 2 out]
          }
          frame True {
            n360 = property on="Waveform_main" class="WFGraph (strict)"("XScale.Maximum"=w490, "XScale.Minimum"=w489) -> ()  [unwired: 2 in, 2 out]
          }
        }
      }
      event "Center": Value Change {
        n361 = event-data() -> ()  [unwired: 1 in, 6 out]
        n362 = property on="Waveform_main" class="WFGraph (strict)"() -> ("XScale.Maximum"=w495:dbl, "XScale.Minimum"=w494:dbl)  [unwired: 2 in, 2 out]
        n363 = Add(x=w495, y=w494) -> (x+y=w493:dbl)
        n364 = Divide(x=w493, y=2.0) -> (x/y=w491:dbl)
        n365 = property on="Waveform_main" class="WFGraph (strict)" props=["Value", "Active Cursor", "Cursor", "Cursor X"]("Active Cursor"=u32 1, "Cursor.Cursor X"=w491) -> (error out=w496:errorcluster)  [unwired: 2 in, 2 out]
        n366 = property on="Waveform_main" class="WFGraph (strict)" props=["CrsrList", "Active Cursor", "Cursor", "Cursor X"](error in=w496, "Active Cursor"=u32 0, "Cursor.Cursor X"=w491) -> ()  [unwired: 1 in, 3 out]
      }
      event "stop": Value Change {
        n367 = event-data() -> ()  [unwired: 1 in, 6 out]
        n368 = flat-sequence {
          tunnel: [w503] -> w499
          tunnel: w499 -> [w512]
          frame #0 {
            n369 = local write "Task out"(refnum<k21> "Stop" ("Task out")) -> ()
          }
          frame #1 {
            n370 = local read "USB"() -> (w511:tag)
            n371 = local read "Task out"() -> (w506:refnum<k21>)
            n372 = call "uA_daq_Set_Relay_internal_power_on_off_from_baterry.vi"("Power ON/OFF DUT"=enum16{"Power ON DUT", "Power OFF DUT"}."Power OFF DUT", "USB DAQ"=w511) -> ("error out"=w502:errorcluster)  [unwired: 9 in]
            n373 = call <vilib>:"DAQmx Stop Task.vi"("task/channels in"=w506, "error in"=w502) -> ("task out"=w501:refnum<k21>, "error out"=w504:errorcluster)  [unwired: 12 in]
            n374 = call <vilib>:"DAQmx Clear Task.vi"("task in"=w501, "error in"=w504) -> ("error out"=w505:errorcluster)  [unwired: 13 in]
            n375 = local read "USB"() -> (w509:tag)
            n376 = call <vilib>:"Clear Errors.vi"("error in (no error)"=w505) -> ("error out"=w508:errorcluster)  [unwired: 5 in, 1 out]
            n377 = call "uA_daq_ON_OFF_LED_Measure.vi"("error in"=w508, "LED_meas"=FALSE ("Boolean"), "USB"=w509) -> ("error out"=w503:errorcluster)  [unwired: 8 in]
          }
          frame #2 {
            n378 = local read "Ver"() -> (w513:string)
            n379 = call <vilib>:"Clear Errors.vi"("error in (no error)"=w512) -> ()  [unwired: 5 in, 2 out]
            n380 = Empty String/Path?(string/path=w513) -> (empty?=w514:bool)
            n381 = case shown="False" w514 {
              frame True {
              }
              frame False {
                n382 = Quit LabVIEW(quit? (T)=TRUE) -> ()
              }
            }
          }
          frame #3 {
            n383 = Stop(stop? (T)=TRUE) -> ()
          }
        }
      }
      event "Save": Value Change {
        n384 = event-data() -> ()  [unwired: 1 in, 6 out]
        n385 = local read "Waveform_main"() -> (w518:waveform(sgl))
        n386 = call "File Dialog"("pattern (all files)"="*.dlog", "pattern label"="datalog") -> ("selected path"=w521:path)  [unwired: 10 in, 3 out]
        n387 = call-poly <vilib>:"Write Waveforms to File.vi"("append to file? (new file:F)"=FALSE, "waveform"=w518, "file path (dialog if empty)"=w521) -> ()  [unwired: 7 in, 2 out]
      }
      event "Load": Value Change {
        (unwired) FALSE ("append to file? (new file:F)")
        n388 = event-data() -> ()  [unwired: 1 in, 6 out]
        n389 = call "File Dialog3"("pattern (all files)"="*.dlog", "pattern label"="datalog") -> ("selected path"=w525:path)  [unwired: 10 in, 3 out]
        n390 = call-poly <vilib>:"Read Waveforms from File.vi"("file path (dialog if empty)"=w525) -> ("first waveform in record"=w522:waveform(dbl))  [unwired: 5 in, 3 out]
        n391 = local write "Waveform_main"(w522) -> ()
      }
      event "Take Picture": Value Change {
        n392 = event-data() -> ()  [unwired: 1 in, 6 out]
        n393 = call <vilib>:"Application Directory.vi"() -> ("Application Directory"=w527:path)
        n394 = control-ref of="This VI"() -> (w531:refnum<vi>)
        n395 = call "File Dialog2"("start path"=w527, "pattern (all files)"="*.jpg", "pattern label"="*.jpg") -> ("selected path"=w533:path, "error out"=w530:errorcluster)  [unwired: 9 in, 2 out]
        n396 = invoke on="Invoke Node" class="VI" method="FP.Get Image"(reference=w531, "image depth"=enum32{"File", "Clipboard"}."File" ("Target")) -> ("image data"=w532:T9)  [unwired: 4 in, 5 out]
        n397 = call <vilib>:"Clear Errors.vi"("error in (no error)"=w530) -> ()  [unwired: 5 in, 2 out]
        n398 = call <vilib>:"Write JPEG File.vi"("image data"=w532, "path to JPEG file"=w533) -> ()  [unwired: 8 in, 2 out]
      }
      event "Save setting": Value Change {
        w555 = "SETTING" ("section")
        n399 = event-data() -> ()  [unwired: 1 in, 6 out]
        n400 = call <vilib>:"Application Directory.vi"() -> ("Application Directory"=w560:path)
        n401 = local read "Range - Shunts"() -> (w548:T2)
        n402 = Build Path(base path=w560, name or relative path="Setting.cfg") -> (appended path=w558:path)
        n403 = local read "Vout  - Vbat profile"() -> (w545:enum16{"3.8VDC", "2.9VDC", "By Pass", "4.0VDC"})
        n404 = call <vilib>:"Open Config Data.vi"("create file if necessary (T)"=TRUE, "configuration file path"=w558) -> ("error out"=w534:errorcluster, "refnum"=w556:T5)  [unwired: 7 in, 1 out]
        n405 = local read "Profile"() -> (w547:enum16{"SAM", "DIANA", "Hi-POWER", "Other..."})
        n406 = call-poly <vilib>:"Write Key.vi"("section"=w555, "error in (no error)"=w534, "value"=w548, "key"="Range - Shunts", "refnum"=w556) -> ("error out"=w535:errorcluster, "refnum out"=w553:T5)  [unwired: 4 in, 1 out]
        n407 = local read "Internal PW"() -> (w543:bool)
        n408 = call-poly <vilib>:"Write Key.vi"("section"=w555, "error in (no error)"=w535, "value"=w547, "key"="Profile", "refnum"=w553) -> ("error out"=w536:errorcluster, "refnum out"=w554:T5)  [unwired: 4 in, 1 out]
        n409 = local read "bypass Shunt"() -> (w541:bool)
        n410 = call-poly <vilib>:"Write Key.vi"("section"=w555, "error in (no error)"=w536, "value"=w545, "key"="Vout  - Vbat profile", "refnum"=w554) -> ("error out"=w537:errorcluster, "refnum out"=w552:T5)  [unwired: 4 in, 1 out]
        n411 = call-poly <vilib>:"Write Key.vi"("section"=w555, "error in (no error)"=w537, "value"=w543, "key"="Internal PW", "refnum"=w552) -> ("error out"=w538:errorcluster, "refnum out"=w551:T5)  [unwired: 4 in, 1 out]
        n412 = call-poly <vilib>:"Write Key.vi"("section"=w555, "error in (no error)"=w538, "value"=w541, "key"="bypass Shunt", "refnum"=w551) -> ("error out"=w539:errorcluster, "refnum out"=w540:T5)  [unwired: 4 in, 1 out]
        n413 = call <vilib>:"Close Config Data.vi"("error in (no error)"=w539, "refnum"=w540) -> ()  [unwired: 8 in, 2 out]
      }
    }
  }
  n414 = while {
    tunnel: w4 -> [w570]
    tunnel: [w569] -> w7
    shift-right: [w565] -> w6
    shift-left: w5 -> [w567]
    stop <- FALSE ("stop (F)") stop-if-true
    n415 = local read "Range - Shunts"() -> (w564:T2)
    n416 = local read "Samples"() -> (w561:i32)
    n417 = Equal?(x=w567, y=refnum<k21> "Stop") -> (x = y?=w563:bool)
    n418 = case shown="True" w563 {
      tunnel: w570 -> [w573 w581]
      tunnel: [w573 w580] -> w569
      tunnel: w567 -> [_ w577]
      tunnel: [w572 w579] -> w565
      tunnel: w564 -> [_ w578]
      tunnel: refnum<k21> refnum ("task out") -> [_ w575]
      tunnel: w561 -> [_ w574]
      frame True {
        n419 = Wait (ms)(milliseconds to wait=u32 100) -> ()  [unwired: 1 out]
        n420 = local read "Task out"() -> (w572:refnum<k21>)
      }
      frame False {
        n421 = Not Equal?(x=w577, y=w575) -> (x != y?=w576:bool)
        n422 = case shown="True" w576 {
          tunnel: w581 -> [w583 w589]
          tunnel: [w583 w588] -> w580
          tunnel: w577 -> [_ w587]
          tunnel: [w582 w586] -> w579
          tunnel: w578 -> [_ w585]
          tunnel: w574 -> [_ w584]
          frame False {
            n423 = local read "Task out"() -> (w582:refnum<k21>)
          }
          frame True {
            n424 = case shown="\"mA Range Rs = 1ohm\"" w585 {
              tunnel: w589 -> [w596 w607 w618 w629]
              tunnel: [w595 w606 w617 w628] -> w588
              tunnel: w587 -> [w594 w605 w616 w627]
              tunnel: [w593 w604 w615 w626] -> w586
              tunnel: w584 -> [w590 w601 w612 w623]
              frame "mA Range Rs = 1ohm" {
                n425 = call "DAQ_ADC_Max_Sample_Rate_For_USB_6001.vi"("number of samples per channel"=w590, "Refnum in"=w594) -> ("error out"=w592:errorcluster, "data"=w591:waveform(dbl))  [unwired: 8 in]
                n426 = case shown="No Error" w592 {
                  selector: w592 -> [_ w600]
                  tunnel: w596 -> [w599 _]
                  tunnel: [w598 _] -> w595
                  tunnel: w591 -> [w597 _]
                  frame No Error {
                    n427 = Enqueue Element(queue=w599, element=w597) -> (queue out=w598:refnum<queue>)  [unwired: 2 in, 2 out]
                  }
                  frame Error {
                    n428 = call <vilib>:"Clear Errors.vi"("error in (no error)"=w600) -> ()  [unwired: 5 in, 2 out]
                  }
                }
                n429 = local read "Task out"() -> (w593:refnum<k21>)
              }
              frame "mA Range Rs = 1ohm - X2" {
                n430 = call "DAQ_ADC_Max_Sample_Rate_For_USB_6001.vi"("number of samples per channel"=w601, "Refnum in"=w605) -> ("error out"=w603:errorcluster, "data"=w602:waveform(dbl))  [unwired: 8 in]
                n431 = case shown="No Error" w603 {
                  selector: w603 -> [_ w611]
                  tunnel: w607 -> [w610 _]
                  tunnel: [w609 _] -> w606
                  tunnel: w602 -> [w608 _]
                  frame No Error {
                    n432 = Enqueue Element(queue=w610, element=w608) -> (queue out=w609:refnum<queue>)  [unwired: 2 in, 2 out]
                  }
                  frame Error {
                    n433 = call <vilib>:"Clear Errors.vi"("error in (no error)"=w611) -> ()  [unwired: 5 in, 2 out]
                  }
                }
                n434 = local read "Task out"() -> (w604:refnum<k21>)
              }
              frame "mA Range Rs = 3.3ohm" {
                n435 = call "DAQ_ADC_Max_Sample_Rate_For_USB_6001.vi"("number of samples per channel"=w612, "Refnum in"=w616) -> ("error out"=w614:errorcluster, "data"=w613:waveform(dbl))  [unwired: 8 in]
                n436 = case shown="No Error" w614 {
                  selector: w614 -> [_ w622]
                  tunnel: w618 -> [w621 _]
                  tunnel: [w620 _] -> w617
                  tunnel: w613 -> [w619 _]
                  frame No Error {
                    n437 = Enqueue Element(queue=w621, element=w619) -> (queue out=w620:refnum<queue>)  [unwired: 2 in, 2 out]
                  }
                  frame Error {
                    n438 = call <vilib>:"Clear Errors.vi"("error in (no error)"=w622) -> ()  [unwired: 5 in, 2 out]
                  }
                }
                n439 = local read "Task out"() -> (w615:refnum<k21>)
              }
              frame "uA Range  Rs = 3.3ohm" {
                n440 = call "DAQ_ADC_Max_Sample_Rate_For_USB_6001.vi"("number of samples per channel"=w623, "Refnum in"=w627) -> ("error out"=w625:errorcluster, "data"=w624:waveform(dbl))  [unwired: 8 in]
                n441 = case shown="No Error" w625 {
                  selector: w625 -> [_ w633]
                  tunnel: w629 -> [w632 _]
                  tunnel: [w631 _] -> w628
                  tunnel: w624 -> [w630 _]
                  frame No Error {
                    n442 = Enqueue Element(queue=w632, element=w630) -> (queue out=w631:refnum<queue>)  [unwired: 2 in, 2 out]
                  }
                  frame Error {
                    n443 = call <vilib>:"Clear Errors.vi"("error in (no error)"=w633) -> ()  [unwired: 5 in, 2 out]
                  }
                }
                n444 = local read "Task out"() -> (w626:refnum<k21>)
              }
            }
          }
        }
      }
    }
  }
  n445 = while {
    tunnel: w4 -> [w641]
    tunnel: w1 -> [w636]
    stop <- FALSE stop-if-true
    n446 = property on="Ext PW Vol Monitor" class="Bool (strict)"() -> ("Value"=w647:bool)  [unwired: 2 in, 2 out]
    n447 = local read "Clear"() -> (w650:bool)
    n448 = property on="Range - Shunts" class="Enum (strict)"() -> ("Value"=w645:T2)  [unwired: 2 in, 2 out]
    n449 = Get Queue Status(queue=w641) -> (queue out=w638:refnum<queue>, error out=w642:errorcluster, # elements in queue=w640:i32)  [unwired: 2 in, 5 out]
    n450 = Dequeue Element(queue=w641, error in (no error)=w642) -> (element=w646:waveform(sgl))  [unwired: 1 in, 3 out]
    n451 = case shown="False" w650 {
      tunnel: [waveform(sgl) {"t0"=timestamp(0 s since 1904-01-01), "dt"=1.0, "Y"=[]} ("Waveform_main") w703] -> w649
      tunnel: w636 -> [_ w701]
      tunnel: [FALSE w700] -> w635
      frame True {
      }
      frame False {
        n452 = local read "Waveform_main"() -> (w703:waveform(sgl))
        n453 = Unbundle By Name(w703) -> ("Y"=w702:sgl[])
        n454 = Array Size(array=w702) -> (size(s)=w699:i32)
        n455 = Greater Or Equal?(x=w699, y=w701) -> (x >= y?=w700:bool)
        n456 = call "Convert  Sample to second.vi"("samples collected"=w699) -> ()  [unwired: 7 in, 4 out]
      }
    }
    n457 = Greater?(x=w640, y=100) -> (0:w637:bool)
    n458 = case shown="\"mA Range Rs = 1ohm\"" w645 {
      tunnel: w646 -> [w656 w660 w664 w668]
      tunnel: [w653 w657 w661 w665] -> w644
      frame "mA Range Rs = 3.3ohm" {
        (unwired) 0.0 ("uA_bank0")
        n459 = call-poly <vilib>:"Basic Averaged DC-RMS.vi"("signal in"=w656) -> ("RMS value"=w654:dbl)  [unwired: 7 in, 3 out]
        n460 = Greater?(x=w654, y=3.5) -> (0:w653:bool)
      }
      frame "uA Range  Rs = 3.3ohm" {
        n461 = call-poly <vilib>:"Basic Averaged DC-RMS.vi"("signal in"=w660) -> ("RMS value"=w658:dbl)  [unwired: 7 in, 3 out]
        n462 = Greater?(x=w658, y=3.5) -> (0:w657:bool)
      }
      frame "mA Range Rs = 1ohm" {
        (unwired) 0.0 ("uA_bank0")
        n463 = call-poly <vilib>:"Basic Averaged DC-RMS.vi"("signal in"=w664) -> ("RMS value"=w662:dbl)  [unwired: 7 in, 3 out]
        n464 = Greater?(x=w662, y=4.0) -> (0:w661:bool)
      }
      frame "mA Range Rs = 1ohm - X2" {
        (unwired) 0.0 ("uA_bank0")
        n465 = call-poly <vilib>:"Basic Averaged DC-RMS.vi"("signal in"=w668) -> ("RMS value"=w666:dbl)  [unwired: 7 in, 3 out]
        n466 = Greater?(x=w666, y=2.0) -> (0:w665:bool)
      }
    }
    n467 = case shown="True" w637 {
      tunnel: w638 -> [_ w652]
      frame False {
      }
      frame True {
        n468 = Flush Queue(queue=w652) -> ()  [unwired: 1 in, 3 out]
      }
    }
    n469 = case shown="True" w647 {
      tunnel: w646 -> [w676 w685]
      tunnel: [w676 w684] -> w634
      tunnel: w644 -> [_ w682]
      tunnel: [FALSE w682] -> w643
      frame True {
        n470 = Unbundle By Name(w676) -> ("Y"=w675:sgl[])
        n471 = Add Array Elements(numeric array=w676) -> (sum=w673:sgl)
        n472 = Array Size(array=w675) -> (size(s)=w674:i32)
        n473 = Divide(x=w673, y=w674) -> (x/y=w670:sgl)
        n474 = Greater?(x=w670, y=6) -> (0:w672:bool)
        n475 = case shown="True" w672 {
          frame False {
          }
          frame True {
            n476 = property on="Internal PW" class="Bool (strict)"("Value"=TRUE ("Internal PW")) -> ()  [unwired: 2 in, 2 out]
            n477 = local read "USB"() -> (w679:tag)
            n478 = call "uA_daq_switch_external_internal_pw_source.vi"("USB DAQ"=w679, "Ex/Int PW"=T6."External PW Source") -> ()  [unwired: 9 in, 1 out]
          }
        }
      }
      frame False {
        n479 = property on="Range - Shunts" class="Enum (strict)"() -> ("Value"=w683:T2)  [unwired: 2 in, 2 out]
        n480 = local read "uA_bank0"() -> (w681:dbl)
        n481 = local read "mARange"() -> (w680:dbl)
        n482 = call "uA_daq_gain_caculator.vi"("Waveform Chart in"=w685, "Calib_value_ uA"=w681, "Calib_mA"=w680, "Range - Shunts"=w683) -> ("Waveform out"=w684:waveform(dbl))  [unwired: 11 in]
      }
    }
    n483 = local read "Measure"() -> (w648:bool)
    n484 = case shown="False" w635 {
      tunnel: w634 -> [_ w690]
      tunnel: w649 -> [_ w689]
      tunnel: w648 -> [w686 w688]
      frame True {
        n485 = case shown="True" w686 {
          frame False {
          }
          frame True {
            n486 = call "Display Message to User4"() -> ()  [unwired: 10 in, 2 out]
          }
        }
        n487 = local write "Measure"(FALSE ("Measure")) -> ()
      }
      frame False {
        n488 = case shown="True" w688 {
          tunnel: w690 -> [_ w692]
          tunnel: w689 -> [_ w694]
          frame False {
          }
          frame True {
            n489 = call "WDT Append Waveforms SGL.vi"("waveform B"=w694, "waveform A"=w692) -> ("waveform out"=→"Waveform_main":waveform(sgl))  [unwired: 8 in, 1 out]
            n490 = local read "Waveform_main"() -> (w695:waveform(sgl))
            n491 = property on="Waveform_main" class="WFGraph (strict)"() -> ("CrsrList"=w696:T8)  [unwired: 2 in, 2 out]
            n492 = call "uA_daq_capture_small_curr_waveform.vi"("CrsrList"=w696, "Waveform_main"=w695) -> ("Numeric"=→"Average (uA)":sgl)  [unwired: 9 in]
          }
        }
      }
    }
    n493 = property on="out_range" class="Bool (strict)"("Visible"=w643) -> ()  [unwired: 2 in, 2 out]
  }
  n494 = Release Queue(queue=w7) -> ()  [unwired: 2 in, 3 out]
  n495 = call <vilib>:"DAQmx Clear Task.vi"("task in"=w6) -> ()  [unwired: 14 in, 1 out]
